vi "graph2.vi"(11 "replay":bool) -> (0 "path_size":i32, 3 "XY Graph":cluster{"Y":dbl[], "Y":dbl[]}[](graph)=[{"Y"=[-25.865695246715575, -25.865695246715575, -25.865695246715575], "Y"=[59.163033466791006, 59.163033466791006, 59.163033466791006]}, {"Y"=[0.85, 0.95, 0.95, 0.6, 0.6, 0.85, 0.85, -0.85, -0.85, -0.95, -0.95, -0.6, -0.6, -0.85, -0.6, -0.6, -0.85, -0.85, 0.85, 0.85], "Y"=[-0.6, -0.6, -1.4, -1.4, -0.6, -0.6, 2.4, 2.4, -0.6, -0.6, -1.4, -1.4, -0.6, -0.6, -0.6, -1.4, -1.4, -1.6, -1.6, -1.4]}, {"Y"=[-25.865695246715575], "Y"=[59.163033466791006]}, {"Y"=[], "Y"=[]}, {"Y"=array[926 elements], "Y"=array[926 elements]}, {"Y"=[nan, nan], "Y"=[nan, nan]}, {"Y"=[-25.865695246715575], "Y"=[59.163033466791006]}, {"Y"=[], "Y"=[]}, {"Y"=[], "Y"=[]}, {"Y"=[0.0], "Y"=[0.0]}, {"Y"=[], "Y"=[]}, {"Y"=[], "Y"=[]}, {"Y"=[691.7888277244315, 691.8377331659157, 691.8864790442867, 691.9350679862869, 691.9835025898547, 692.0317854247338, 692.079919033068, 692.1279059299806, 692.1757486041453, 692.2234495183519, 692.2710111100497, 692.3184357918904, 692.365725952261, 692.412883955801, 692.4599121439145, 692.5068128352747, 692.5535883263143, 692.6002408917145, 692.6467727848759, 692.6931862383941, 692.7394834645125, 692.785666655583, 692.8317379845035, 692.8776996051629, 692.9235536528688, 692.969302244769, 693.0149474802747, 693.060491441465, 693.1059361934975, 693.151283785001, 693.196536248471, 693.2416956006535, 693.2867638429291, 693.3317429616844, 693.3766349286853, 693.4214417014377, 693.4661652235502, 693.5108074250859, 693.5553702229134, 693.5998555210545, 693.6442652110193, 693.6886011721464, 693.7328652719325, 693.7770593663641, 693.8211853002351, 693.8652449074733, 693.9092400114525, 693.9531724253069, 693.9970439522381, 694.0408563858227, 694.0846115103164, 694.1283111009493, 694.1719569242241, 694.2155507382114, 694.259094292835, 694.3025893301664, 694.3460375847027, 694.3894407836557, 694.4328006472265, 694.476118888889, 694.5193972156585, 694.5626373283712, 694.6058409219545, 694.6490096856918, 694.6921453034947, 694.7352494541701, 694.7783238116778, 694.8213700453995, 694.8643898203949, 694.9073847976673, 694.9503566344149, 694.9933069842926, 695.0362374976652, 695.079149821865, 695.1220456014439, 695.1649264784243, 695.2077940925565, 695.2506500815632, 695.2934960813969, 695.3363337264864, 695.3791646499868, 695.4219904840265, 695.464812859962, 695.5076334086223, 695.5504537605557, 695.5932755462828, 695.6361003965429, 695.6789299425405, 695.7217658161954, 695.7646096503946, 695.807463079234, 695.8503277382761, 695.8932052647941, 695.9360972980251], "Y"=[-402.1714380892973, -402.2324443015287, -402.29325146963055, -402.3538628702814, -402.4142817442331, -402.47451129706894, -402.53455469993827, -402.5944150902866, -402.6540955725668, -402.71359921893855, -402.7729290699565, -402.832088135239, -402.8910793941361, -402.9499057963747, -403.00857026269705, -403.0670756854909, -403.12542492940014, -403.18362083193375, -403.24166620405737, -403.2995638307791, -403.3573164717253, -403.4149268617041, -403.4723977112591, -403.5297317072198, -403.58693151323575, -403.64399977030746, -403.7009390973042, -403.7577520914824, -403.81444132898264, -403.8710093653304, -403.9274587359257, -403.98379195652205, -404.0400115237071, -404.09611991536156, -404.1521195911291, -404.2080129928654, -404.2638025450895, -404.3194906554251, -404.375079715037, -404.4305720990579, -404.4859701670225, -404.5412762632748, -404.596492717394, -404.6516218445924, -404.70666594612766, -404.76162730969963, -404.81650820984265, -404.87131090831787, -404.9260376544974, -404.98069068574665, -405.0352722278018, -405.0897844951429, -405.14422969136206, -405.19861000952994, -405.2529276325616, -405.30718473357007, -405.3613834762236, -405.41552601510165, -405.46961449603776, -405.52365105647283, -405.5776378257941, -405.6315769256789, -405.685470470432, -405.7393205673213, -405.7931293169138, -405.84689881340205, -405.90063114494075, -405.9543283939694, -406.0079926375368, -406.0616259476311, -406.11523039149404, -406.1688080319476, -406.2223609277105, -406.2758911337184, -406.3294007014348, -406.38289167917463, -406.4363661124128, -406.4898260440976, -406.54327351496966, -406.5967105638653, -406.65013922803496, -406.70356154344927, -406.75697954511423, -406.8103952673769, -406.8638107442369, -406.9172280096572, -406.97064909787343, -407.0240760437018, -407.0775108828543, -407.1309556522436, -407.18441239029335, -407.23788313725817, -407.2913699355226, -407.3448748299264]}, {"Y"=[], "Y"=[]}, {"Y"=[-0.152017305614708], "Y"=[0.5451838106381299]}])   [LabVIEW 2015]
uses:
  G_NAV.vi
  G_PATH.vi
  G_VEH.vi
  G_SEN.vi
  G_LCM.vi
  <vilib>/Analysis/Matrix/Datatypes/RealMatrix.ctl
  <vilib>/Analysis/Matrix/NI_Matrix.lvlib
  <vilib>/Analysis/NI_AALBase.lvlib
  <vilib>/Analysis/baseanly.llb/Real A x B.vi
panel:
  out "x 17":dbl[](array[numeric])=[-13.0, -13.0, -13.0, -13.0, -13.0, -13.0, -13.0, -13.0, -13.0, -13.0, -13.0, -13.0, -13.0, -13.0, -13.0, -13.0, -13.0, -13.0, -13.0, -13.0, -13.0, -13.0, -13.0, -13.0, -13.0, -13.25, -13.25, -13.25, -13.25, -13.25, -13.25, -13.25, -13.25, -13.25, -13.25, -13.25, -13.25, -13.25, -13.25, -13.25, -13.25, -13.25, -13.25, -13.25, -13.25, -13.5, -13.25, -13.25, -13.25, -13.5, -13.5, -13.25, -13.5, -13.5, -13.5, -13.5, -13.5, -13.25, -13.5, -13.5, -13.75, -13.5, -13.5, -13.25, -13.75, -13.75, -13.5, -13.5, -13.5, -14.0, -14.0, -14.0, -13.75, -13.75, -13.75, -13.75, -1.0, -1.0, -0.75, -0.75, -0.75, -0.5, -0.5, -0.5, -0.25, -0.25, -0.25, -0.25, 0.0, 0.0, 0.0, 0.0, 0.0, 0.25, 0.25, 0.25, 0.25, 0.25, 0.5, 0.5, 0.5, 0.5, 0.75, 0.75, 0.75, 1.0, 1.0, 1.25, 1.25, 1.25, 1.5, 1.5]
  out "y 17":dbl[](array[numeric])=[0.0, 0.25, 0.5, 0.75, 1.0, 1.25, 1.25, 1.5, 1.75, 2.0, 2.25, 2.5, 2.75, 3.0, 3.25, 3.5, 3.75, 4.0, 4.25, 4.5, 4.75, 5.0, 5.25, 5.5, 5.75, 6.0, 6.5, 6.75, 7.0, 7.25, 7.5, 8.0, 8.25, 8.5, 9.0, 9.25, 9.5, 10.0, 10.25, 10.75, 11.25, 11.5, 12.0, 12.5, 13.0, 13.5, 13.75, 14.25, 14.75, 15.5, 16.0, 16.5, 17.25, 18.0, 18.5, 19.5, 20.0, 20.5, 21.75, 22.25, 23.75, 24.5, 25.25, 26.25, 28.25, 29.25, 30.5, 31.75, 33.25, 36.5, 38.25, 40.5, 42.75, 45.25, 48.25, 51.5, 4.25, 4.0, 4.0, 4.0, 3.75, 3.75, 3.75, 3.5, 3.5, 3.5, 3.25, 3.25, 3.25, 3.25, 3.25, 3.25, 3.0, 3.0, 3.0, 3.0, 3.0, 2.75, 3.0, 3.0, 3.0, 3.25, 3.25, 3.25, 3.5, 3.5, 3.5, 3.75, 3.75, 4.0, 4.0, 4.25]
  out "x 16":dbl[](array[numeric])=[-13.0, -13.0, -13.0, -13.0, -13.0, -13.0, -13.0, -13.0, -13.0, -13.0, -13.0, -13.0, -13.0, -13.0, -13.0, -13.0, -13.0, -13.0, -13.0, -13.0, -13.0, -13.0, -13.0, -13.0, -13.0, -13.25, -13.25, -13.25, -13.25, -13.25, -13.25, -13.25, -13.25, -13.25, -13.25, -13.25, -13.25, -13.25, -13.25, -13.25, -13.25, -13.25, -13.25, -13.25, -13.25, -13.5, -13.25, -13.25, -13.25, -13.5, -13.5, -13.25, -13.5, -13.5, -13.5, -13.5, -13.5, -13.25, -13.5, -13.5, -13.75, -13.5, -13.5, -13.25, -13.75, -13.75, -13.5, -13.5, -13.5, -14.0, -14.0, -14.0, -13.75, -13.75, -13.75, -13.75, -1.0, -1.0, -0.75, -0.75, -0.75, -0.5, -0.5, -0.5, -0.25, -0.25, -0.25, -0.25, 0.0, 0.0, 0.0, 0.0, 0.0, 0.25, 0.25, 0.25, 0.25, 0.25, 0.5, 0.5, 0.5, 0.5, 0.75, 0.75, 0.75, 1.0, 1.0, 1.25, 1.25, 1.25, 1.5, 1.5]
  out "y 16":dbl[](array[numeric])=[0.0, 0.25, 0.5, 0.75, 1.0, 1.25, 1.25, 1.5, 1.75, 2.0, 2.25, 2.5, 2.75, 3.0, 3.25, 3.5, 3.75, 4.0, 4.25, 4.5, 4.75, 5.0, 5.25, 5.5, 5.75, 6.0, 6.5, 6.75, 7.0, 7.25, 7.5, 8.0, 8.25, 8.5, 9.0, 9.25, 9.5, 10.0, 10.25, 10.75, 11.25, 11.5, 12.0, 12.5, 13.0, 13.5, 13.75, 14.25, 14.75, 15.5, 16.0, 16.5, 17.25, 18.0, 18.5, 19.5, 20.0, 20.5, 21.75, 22.25, 23.75, 24.5, 25.25, 26.25, 28.25, 29.25, 30.5, 31.75, 33.25, 36.5, 38.25, 40.5, 42.75, 45.25, 48.25, 51.5, 4.25, 4.0, 4.0, 4.0, 3.75, 3.75, 3.75, 3.5, 3.5, 3.5, 3.25, 3.25, 3.25, 3.25, 3.25, 3.25, 3.0, 3.0, 3.0, 3.0, 3.0, 2.75, 3.0, 3.0, 3.0, 3.25, 3.25, 3.25, 3.5, 3.5, 3.5, 3.75, 3.75, 4.0, 4.0, 4.25]
  out "M6006":T1={"GPSTime"=22892800.0, "attitude[2]"=-0.6123908, "lcc[0]"=-970.47205, "lcc[1]"=200.52362, "heading_GPS"=-0.6106907} {"GPSTime" format="%#_6f"}
  out "y 5":dbl[](array[numeric])
  out "x 5":dbl[](array[numeric])
  out "y 4":dbl[](array[numeric])
  out "x 4":dbl[](array[numeric])
  out "y 6":dbl[](array[numeric])
  out "x 6":dbl[](array[numeric])
  out "x 14":dbl[](array[numeric])
  out "y 14":dbl[](array[numeric])
  out "y 10":dbl[](array[numeric])
  out "x 10":dbl[](array[numeric])
  out "y 1":dbl[](array[numeric])
  out "x 1":dbl[](array[numeric])
  out "y 15":dbl[](array[numeric])=[0.0, 0.25, 0.5, 0.75, 1.0, 1.25, 1.25, 1.5, 1.75, 2.0, 2.25, 2.5, 2.75, 3.0, 3.25, 3.5, 3.75, 4.0, 4.25, 4.5, 4.75, 5.0, 5.25, 5.5, 5.75, 6.0, 6.5, 6.75, 7.0, 7.25, 7.5, 8.0, 8.25, 8.5, 9.0, 9.25, 9.5, 10.0, 10.25, 10.75, 11.25, 11.5, 12.0, 12.5, 13.0, 13.5, 13.75, 14.25, 14.75, 15.5, 16.0, 16.5, 17.25, 18.0, 18.5, 19.5, 20.0, 20.5, 21.75, 22.25, 23.75, 24.5, 25.25, 26.25, 28.25, 29.25, 30.5, 31.75, 33.25, 36.5, 38.25, 40.5, 42.75, 45.25, 48.25, 51.5, 4.25, 4.0, 4.0, 4.0, 3.75, 3.75, 3.75, 3.5, 3.5, 3.5, 3.25, 3.25, 3.25, 3.25, 3.25, 3.25, 3.0, 3.0, 3.0, 3.0, 3.0, 2.75, 3.0, 3.0, 3.0, 3.25, 3.25, 3.25, 3.5, 3.5, 3.5, 3.75, 3.75, 4.0, 4.0, 4.25]
  out "x 15":dbl[](array[numeric])=[-13.0, -13.0, -13.0, -13.0, -13.0, -13.0, -13.0, -13.0, -13.0, -13.0, -13.0, -13.0, -13.0, -13.0, -13.0, -13.0, -13.0, -13.0, -13.0, -13.0, -13.0, -13.0, -13.0, -13.0, -13.0, -13.25, -13.25, -13.25, -13.25, -13.25, -13.25, -13.25, -13.25, -13.25, -13.25, -13.25, -13.25, -13.25, -13.25, -13.25, -13.25, -13.25, -13.25, -13.25, -13.25, -13.5, -13.25, -13.25, -13.25, -13.5, -13.5, -13.25, -13.5, -13.5, -13.5, -13.5, -13.5, -13.25, -13.5, -13.5, -13.75, -13.5, -13.5, -13.25, -13.75, -13.75, -13.5, -13.5, -13.5, -14.0, -14.0, -14.0, -13.75, -13.75, -13.75, -13.75, -1.0, -1.0, -0.75, -0.75, -0.75, -0.5, -0.5, -0.5, -0.25, -0.25, -0.25, -0.25, 0.0, 0.0, 0.0, 0.0, 0.0, 0.25, 0.25, 0.25, 0.25, 0.25, 0.5, 0.5, 0.5, 0.5, 0.75, 0.75, 0.75, 1.0, 1.0, 1.25, 1.25, 1.25, 1.5, 1.5]
  out "y 13":dbl[](array[numeric])=[0.0, 0.25, 0.5, 0.75, 1.0, 1.25, 1.25, 1.5, 1.75, 2.0, 2.25, 2.5, 2.75, 3.0, 3.25, 3.5, 3.75, 4.0, 4.25, 4.5, 4.75, 5.0, 5.25, 5.5, 5.75, 6.0, 6.5, 6.75, 7.0, 7.25, 7.5, 8.0, 8.25, 8.5, 9.0, 9.25, 9.5, 10.0, 10.25, 10.75, 11.25, 11.5, 12.0, 12.5, 13.0, 13.5, 13.75, 14.25, 14.75, 15.5, 16.0, 16.5, 17.25, 18.0, 18.5, 19.5, 20.0, 20.5, 21.75, 22.25, 23.75, 24.5, 25.25, 26.25, 28.25, 29.25, 30.5, 31.75, 33.25, 36.5, 38.25, 40.5, 42.75, 45.25, 48.25, 51.5, 4.25, 4.0, 4.0, 4.0, 3.75, 3.75, 3.75, 3.5, 3.5, 3.5, 3.25, 3.25, 3.25, 3.25, 3.25, 3.25, 3.0, 3.0, 3.0, 3.0, 3.0, 2.75, 3.0, 3.0, 3.0, 3.25, 3.25, 3.25, 3.5, 3.5, 3.5, 3.75, 3.75, 4.0, 4.0, 4.25]
  out "x 13":dbl[](array[numeric])=[-13.0, -13.0, -13.0, -13.0, -13.0, -13.0, -13.0, -13.0, -13.0, -13.0, -13.0, -13.0, -13.0, -13.0, -13.0, -13.0, -13.0, -13.0, -13.0, -13.0, -13.0, -13.0, -13.0, -13.0, -13.0, -13.25, -13.25, -13.25, -13.25, -13.25, -13.25, -13.25, -13.25, -13.25, -13.25, -13.25, -13.25, -13.25, -13.25, -13.25, -13.25, -13.25, -13.25, -13.25, -13.25, -13.5, -13.25, -13.25, -13.25, -13.5, -13.5, -13.25, -13.5, -13.5, -13.5, -13.5, -13.5, -13.25, -13.5, -13.5, -13.75, -13.5, -13.5, -13.25, -13.75, -13.75, -13.5, -13.5, -13.5, -14.0, -14.0, -14.0, -13.75, -13.75, -13.75, -13.75, -1.0, -1.0, -0.75, -0.75, -0.75, -0.5, -0.5, -0.5, -0.25, -0.25, -0.25, -0.25, 0.0, 0.0, 0.0, 0.0, 0.0, 0.25, 0.25, 0.25, 0.25, 0.25, 0.5, 0.5, 0.5, 0.5, 0.75, 0.75, 0.75, 1.0, 1.0, 1.25, 1.25, 1.25, 1.5, 1.5]
  out "y 12":dbl[](array[numeric])=[0.0, 0.25, 0.5, 0.75, 1.0, 1.25, 1.25, 1.5, 1.75, 2.0, 2.25, 2.5, 2.75, 3.0, 3.25, 3.5, 3.75, 4.0, 4.25, 4.5, 4.75, 5.0, 5.25, 5.5, 5.75, 6.0, 6.5, 6.75, 7.0, 7.25, 7.5, 8.0, 8.25, 8.5, 9.0, 9.25, 9.5, 10.0, 10.25, 10.75, 11.25, 11.5, 12.0, 12.5, 13.0, 13.5, 13.75, 14.25, 14.75, 15.5, 16.0, 16.5, 17.25, 18.0, 18.5, 19.5, 20.0, 20.5, 21.75, 22.25, 23.75, 24.5, 25.25, 26.25, 28.25, 29.25, 30.5, 31.75, 33.25, 36.5, 38.25, 40.5, 42.75, 45.25, 48.25, 51.5, 4.25, 4.0, 4.0, 4.0, 3.75, 3.75, 3.75, 3.5, 3.5, 3.5, 3.25, 3.25, 3.25, 3.25, 3.25, 3.25, 3.0, 3.0, 3.0, 3.0, 3.0, 2.75, 3.0, 3.0, 3.0, 3.25, 3.25, 3.25, 3.5, 3.5, 3.5, 3.75, 3.75, 4.0, 4.0, 4.25]
  out "x 12":dbl[](array[numeric])=[-13.0, -13.0, -13.0, -13.0, -13.0, -13.0, -13.0, -13.0, -13.0, -13.0, -13.0, -13.0, -13.0, -13.0, -13.0, -13.0, -13.0, -13.0, -13.0, -13.0, -13.0, -13.0, -13.0, -13.0, -13.0, -13.25, -13.25, -13.25, -13.25, -13.25, -13.25, -13.25, -13.25, -13.25, -13.25, -13.25, -13.25, -13.25, -13.25, -13.25, -13.25, -13.25, -13.25, -13.25, -13.25, -13.5, -13.25, -13.25, -13.25, -13.5, -13.5, -13.25, -13.5, -13.5, -13.5, -13.5, -13.5, -13.25, -13.5, -13.5, -13.75, -13.5, -13.5, -13.25, -13.75, -13.75, -13.5, -13.5, -13.5, -14.0, -14.0, -14.0, -13.75, -13.75, -13.75, -13.75, -1.0, -1.0, -0.75, -0.75, -0.75, -0.5, -0.5, -0.5, -0.25, -0.25, -0.25, -0.25, 0.0, 0.0, 0.0, 0.0, 0.0, 0.25, 0.25, 0.25, 0.25, 0.25, 0.5, 0.5, 0.5, 0.5, 0.75, 0.75, 0.75, 1.0, 1.0, 1.25, 1.25, 1.25, 1.5, 1.5]
  out "y 11":dbl[](array[numeric])=[0.0, 0.25, 0.5, 0.75, 1.0, 1.25, 1.25, 1.5, 1.75, 2.0, 2.25, 2.5, 2.75, 3.0, 3.25, 3.5, 3.75, 4.0, 4.25, 4.5, 4.75, 5.0, 5.25, 5.5, 5.75, 6.0, 6.5, 6.75, 7.0, 7.25, 7.5, 8.0, 8.25, 8.5, 9.0, 9.25, 9.5, 10.0, 10.25, 10.75, 11.25, 11.5, 12.0, 12.5, 13.0, 13.5, 13.75, 14.25, 14.75, 15.5, 16.0, 16.5, 17.25, 18.0, 18.5, 19.5, 20.0, 20.5, 21.75, 22.25, 23.75, 24.5, 25.25, 26.25, 28.25, 29.25, 30.5, 31.75, 33.25, 36.5, 38.25, 40.5, 42.75, 45.25, 48.25, 51.5, 4.25, 4.0, 4.0, 4.0, 3.75, 3.75, 3.75, 3.5, 3.5, 3.5, 3.25, 3.25, 3.25, 3.25, 3.25, 3.25, 3.0, 3.0, 3.0, 3.0, 3.0, 2.75, 3.0, 3.0, 3.0, 3.25, 3.25, 3.25, 3.5, 3.5, 3.5, 3.75, 3.75, 4.0, 4.0, 4.25]
  out "x 11":dbl[](array[numeric])=[-13.0, -13.0, -13.0, -13.0, -13.0, -13.0, -13.0, -13.0, -13.0, -13.0, -13.0, -13.0, -13.0, -13.0, -13.0, -13.0, -13.0, -13.0, -13.0, -13.0, -13.0, -13.0, -13.0, -13.0, -13.0, -13.25, -13.25, -13.25, -13.25, -13.25, -13.25, -13.25, -13.25, -13.25, -13.25, -13.25, -13.25, -13.25, -13.25, -13.25, -13.25, -13.25, -13.25, -13.25, -13.25, -13.5, -13.25, -13.25, -13.25, -13.5, -13.5, -13.25, -13.5, -13.5, -13.5, -13.5, -13.5, -13.25, -13.5, -13.5, -13.75, -13.5, -13.5, -13.25, -13.75, -13.75, -13.5, -13.5, -13.5, -14.0, -14.0, -14.0, -13.75, -13.75, -13.75, -13.75, -1.0, -1.0, -0.75, -0.75, -0.75, -0.5, -0.5, -0.5, -0.25, -0.25, -0.25, -0.25, 0.0, 0.0, 0.0, 0.0, 0.0, 0.25, 0.25, 0.25, 0.25, 0.25, 0.5, 0.5, 0.5, 0.5, 0.75, 0.75, 0.75, 1.0, 1.0, 1.25, 1.25, 1.25, 1.5, 1.5]
  out "y 9":dbl[](array[numeric])=[-40.25486400827094, -40.04085960963455, -39.821235299880705, -39.59593792545196, -39.364914332790825, -39.12811136833988, -38.88547587854164, -38.636954709838655, -38.382494708673484, -38.12204272148863, -37.85554559472668, -37.58295017483014, -37.30420330824157, -37.0192518414035, -36.728042620758494, -36.43052249274907, -36.126638303817785, -35.81633690040717, -35.49956512895978, -35.176269835918156, -34.846397867724825, -34.50989607082233, -34.166711291653236, -33.81679037666006, -33.460080172285366, -33.09652752497168, -32.72607928116154, -32.3486822872975, -31.96428338982209, -31.57282943517787, -31.17426726980736, -30.768543740153135, -30.355605692657697, -30.338651341222633, -30.338651341222633, -29.95729378436619, -29.572397676750224, -29.183911226613308, -28.791782642194068, -28.395960131731087, -27.996391903462964, -27.593026165628288, -27.185811126465662, -26.774694994213668, -26.359625977110902, -25.940552283395995, -25.5174221213075, -25.090183699084033, -24.658785224964184, -24.22317490718656, -23.783300953989748, -23.33911157361234, -22.89055497429293, -22.43757936427013, -21.980132951782515, -21.5181639450687, -21.05162055236726, -20.58045098191681, -20.10460344195595, -19.62402614072324, -19.138667286457324, -18.648475087396758, -18.153397751780158, -17.653383487846114, -17.14838050383323, -16.6383370079801, -16.123201208525305, -15.602921313707439, -15.077445531765132, -14.546722070936944, -14.010699139461483, -13.469324945577348, -12.922547697523145, -12.370315603537431, -11.812576871858855, -11.249279710725965, -10.68037232837739, -10.105802933051706, -9.52551973298753, -8.939470936423437, -8.347604751598034, -8.312579060465806, -8.312579060465806, -7.815979397588906, -7.318560473773825, -6.820356240811432, -6.321400650492564, -5.8217276546080905, -5.321371204948849, -4.820365253305692, -4.318743751469474, -3.816540651231034, -3.313789904381253, -2.8105254627109564, -2.3067812780109964, -1.8025913020722415, -1.2979894866855162, -0.7930097836417018, -0.2876861447316371, 0.2179474782538381, 0.7238571335238572, 1.2300088692875666, 1.7363687337541345, 2.2429027751326935, 2.7495770416323975, 3.2563575814623866, 3.763210442831828, 4.270101673949855, 4.776997323025622, 5.283863438268267, 5.79066606788696, 6.297371260090832, 6.803945063089038, 7.310353525090725, 7.816562694305046, 8.322538618941149, 8.82824734720817, 9.333654927315276, 9.532792066869051, 9.532792066869058, 10.032676667529001, 10.532532309358876, 11.032359899557544, 11.53216034532386, 12.03193455385667, 12.53168343235485, 13.03140788801724, 13.531108828042706, 14.030787159630101, 14.530443789978285, 15.030079626286113, 15.529695575752449, 16.029292545576137, 16.52887144295605, 17.028433175091028, 17.527978649179936, 18.02750877242164, 18.527024452014977, 19.026526595158828, 19.526016109052026, 20.025493900893448, 20.52496087788194, 21.02441794721636, 21.523866016095567, 22.023305991718424, 22.522738781283774, 23.022165291990486, 23.521586431037413, 24.021003105623414, 24.520416222947343, 25.01982669020806, 25.51923541460442, 26.018643303335274, 26.518051263599492, 27.017460202595917, 27.51687102752342, 28.016284645580857, 28.515701963967068, 29.01512388988093, 29.51455133052128, 30.013985193087, 30.513426384776935, 31.012875812789932, 31.512334384324856, 32.01180300658057, 32.511282586755925, 33.01077403204978, 33.51027824966099, 34.00979614678842, 34.15163746485512, 34.15163746485511, 34.65085156194158, 35.150114036225105, 35.649423358614406, 36.148778000018126, 36.64817643134495, 37.14761712350358, 37.64709854740265, 38.14661917395086, 38.64617747405689, 39.14577191862942, 39.6454009785771, 40.14506312480863, 40.644756828232666, 41.14448055975791, 41.644232790293024, 42.14401199074667, 42.643816632027544, 43.14364518504432, 43.64349612070567, 44.14336790992027, 44.6432590235968, 45.14316793264393, 45.64309310797034, 46.143033020484694, 46.64298614109569, 47.14295094071199, 47.64292589024228, 48.14290946059522, 48.64290012267951, 49.142896347403784, 49.64289660567677, 50.142899368407114, 50.64290310650349, 51.14290629087459, 51.64290739242908, 52.14290488207564, 52.64289723072293, 53.142882909279656, 53.642860388654476, 54.14282813975608, 54.64278463349311, 55.14272834077427, 55.64265773250823, 56.14257127960367, 56.642467452969264, 57.142344723513695, 57.642201562145615, 58.14203643977374, 58.6418478273067, 59.141634195653204, 59.641394015721914, 60.1411257584215, 60.64082789466066, 61.14049889534806, 61.64013723139237, 62.139741373702265, 62.63930979318643, 63.138840960753534, 63.63833334731226, 64.13778542377129, 64.63719566103929, 65.1365625300249, 65.63588450163687, 66.13516004678382, 66.62661681170006, 66.62661681170006, 67.12576345342403, 67.62478981859165, 68.1236869902195, 68.62244605132406, 69.12105808492187, 69.61951417402948, 70.11780540166339, 70.61592285084015, 71.11385760457627, 71.61160074588827, 72.10914335779272, 72.6064765233061, 73.10359132544497, 73.60047884722584, 74.09713017166524, 74.59353638177971, 75.08968856058576, 75.58557779109994, 76.08119515633875, 76.57653173931875, 77.07157862305642, 77.56632689056836, 78.060767624871, 78.55489190898098, 79.04869082591473, 79.54215545868882, 80.03527689031979, 80.52804620382416, 81.02045448221844, 81.51249280851917, 82.00415226574289, 82.49542393690609, 82.98629890502534, 83.47676825311716, 83.96682306419804, 84.45645442128455, 84.9456534073932, 85.43441110554052, 85.92271859874306, 86.4105669700173, 86.89794730237979, 87.17622393756727, 87.17622393756727, 87.62090998324233, 88.06278904034333, 88.5018353078985, 88.93802298493607, 89.37132627048422, 89.80171936357122, 90.22917646322526, 90.65367176847454, 91.07517947834734, 91.49367379187183, 91.90912890807624, 92.3215190259888, 92.73081834463773, 93.13700106305124, 93.54004138025758, 93.93991349528491, 94.3365916071615, 94.73004991491554, 95.12026261757528, 95.50720391416891, 95.89084800372467, 96.27116908527078, 96.64814135783546, 97.02173902044692, 97.39193627213336, 97.75870731192305, 98.12202633884417, 98.48186755192496, 98.83820515019363, 99.19101333267841, 99.54026629840749, 99.88593824640913, 99.89953643323281, 99.89953643323281, 100.21054094201504, 100.51734678566943, 100.81989169992012, 101.11811342049135, 101.41194968310735, 101.70133822349231, 101.98621677737043, 102.26652308046596, 102.54219486850307, 102.81316987720602, 103.07938584229896, 103.34078049950615, 103.59729158455178, 103.84885683316006, 104.09541398105519, 104.33690076396141, 104.5732549176029, 104.80441417770389, 105.0303162799886, 105.2508989601812, 105.46609995400595, 105.67585699718703, 105.88010782544866, 106.07879017451506, 106.27184178011042, 106.45920037795898, 106.64080370378494, 106.81658949331246, 106.98649548226584, 107.15045940636924, 107.30841900134685, 107.46031200292295, 107.60607614682168, 107.74564916876727, 107.87896880448396, 108.00597278969595, 108.12659886012742, 108.24078475150262, 108.34846819954572, 108.44958693998096, 108.54407870853257, 108.63188124092471, 108.71293227288164, 108.78716954012754, 108.85453077838663, 108.91495372338314, 108.96837611084122, 108.97747618937277, 108.97747618937277, 109.0156550246946, 109.04983247580746, 109.08011123358501, 109.10659398890081, 109.12938343262847, 109.14858225564154, 109.16429314881364, 109.17661880301837, 109.18566190912927, 109.19152515801999, 109.19431124056405, 109.19412284763511, 109.1910626701067, 109.18523339885247, 109.17673772474595, 109.16567833866077, 109.15215793147051, 109.13627919404871, 109.11814481726906, 109.09785749200506, 109.07551990913035, 109.05123475951848, 109.02510473404305, 108.99723252357771, 108.96772081899594, 108.93667231117144, 108.90418969097772, 108.87037564928839, 108.83533287697705, 108.79916406491728, 108.7619719039827, 108.72385908504685, 108.68492829898334, 108.64528223666576, 108.60502358896771, 108.56425504676278, 108.52307930092454, 108.48159904232658, 108.4399169618425, 108.39813575034592, 108.35635809871036, 108.31468669780945, 108.27322423851678, 108.23207341170594, 108.19133690825049, 108.15111741902408, 108.11151763490025, 108.07264024675257, 108.03458794545469, 107.99746342188017, 107.96136936690259, 107.92640847139555, 107.89268342623265, 107.86029692228745, 107.82935165043357, 107.79995030154457, 107.78125898031978, 107.78125898031978, 107.75369240153198, 107.72548456275034, 107.69669916249154, 107.66739989927227, 107.63765047160923, 107.60751457801909, 107.57705591701853, 107.54633818712422, 107.51542508685286, 107.48438031472112, 107.45326756924571, 107.42215054894329, 107.39109295233057, 107.36015847792419, 107.32941082424084, 107.29891368979723, 107.26873077311004, 107.23892577269594, 107.2095623870716, 107.18070431475374, 107.15241525425903, 107.12475890410411, 107.09779896280573, 107.07159912888052, 107.04622310084521, 107.02173457721644, 106.9981972565109, 106.97567483724531, 106.95423101793631, 106.9339294971006, 106.91483397325487, 106.89700814491579, 106.88051571060006, 106.86545285263342, 106.86545285263342, 106.85123591176482, 106.8373215059327, 106.82369194296759, 106.81032953069995, 106.79721657696027, 106.78433538957903, 106.7716682763867, 106.75919754521381, 106.74690550389077, 106.73477446024813, 106.72278672211637, 106.71092459732593, 106.69917039370733, 106.68750641909104, 106.67591498130754, 106.66437838818732, 106.65287894756085, 106.64139896725864, 106.62992075511116, 106.61842661894889, 106.60689886660232, 106.59531980590192, 106.5836717446782, 106.57193699076163, 106.56009785198269, 106.54813663617186, 106.53603565115962, 106.52377720477648, 106.51134360485288, 106.49871715921937, 106.4858801757064, 106.47281496214443, 106.45950382636393, 106.44592907619545, 106.43207301946944, 106.41791796401637, 106.40344621766674, 106.38864008825105, 106.37348188359975, 106.35795391154335, 106.34203847991229, 106.32571789653713, 106.30897446924827, 106.29179050587625, 106.27414831425155, 106.2560637066309]
  out "x 9":dbl[](array[numeric])=[-22.968902627554595, -22.51700484334325, -22.067726202847595, -21.62109147813308, -21.177125441265126, -20.735852864309198, -20.297298519330727, -19.86148717839516, -19.42844361356793, -18.998192596914485, -18.57075890050028, -18.146167296390736, -17.724442556651315, -17.305609453347444, -16.889692758544577, -16.476717244308148, -16.0667076827036, -15.659688845796383, -15.255685505651932, -14.854722434335699, -14.456824403913117, -14.062016186449632, -13.67032255401068, -13.28176827866172, -12.896378132468183, -12.514176887495505, -12.135189315809143, -11.759440189474532, -11.38695428055711, -11.017756361122329, -10.651871203235629, -10.289323578962446, -9.930138260368233, -9.915595940630572, -9.915595940630572, -9.592217431479307, -9.27296664733781, -8.957904003376973, -8.64708991476769, -8.340584796680856, -8.038449064287356, -7.740743132758091, -7.447527417263952, -7.158862332975826, -6.874808295064605, -6.595425718701188, -6.320775019056462, -6.05091661130132, -5.7859109106066535, -5.525818332143363, -5.270699291082332, -5.02061420259445, -4.775623481850621, -4.535787544021732, -4.301166804278667, -4.071821677792334, -3.8478125797336116, -3.6291999252734, -3.4160441295825903, -3.2084056078320766, -3.0063447751927437, -2.809922046835485, -2.619197837931207, -2.4342325636507813, -2.255086639165114, -2.0818204796450988, -1.9144945002616136, -1.7531691161855663, -1.597904742587841, -1.4487617946393383, -1.3058006875109367, -1.1690818363735358, -1.0386656563980352, -0.9146125627553217, -0.796982970616279, -0.6858372951518088, -0.581235951532802, -0.4832393549301528, -0.3919079205147527, -0.30730206345748806, -0.22948219892925836, -0.22511372738602808, -0.22511372738602808, -0.16680067513880384, -0.11507613036628858, -0.06966705231019729, -0.03030040021222455, 0.0032968666859287954, 0.03139778914256819, 0.05427540791599236, 0.07220276376450722, 0.08545289744639678, 0.09429884971998208, 0.09901366134354672, 0.09987037307539658, 0.09714202567383796, 0.0911016598971616, 0.08202231650367428, 0.0701770362516814, 0.055838859899467026, 0.0392808282053517, 0.020775981927619973, 0.0005973618245841139, -0.020981991345463767, -0.043689036824225154, -0.06725073385338684, -0.09139404167465787, -0.11584591952973904, -0.14033332666033183, -0.164583222308123, -0.18832256571482164, -0.21127831612212852, -0.233177432771738, -0.25374687490535136, -0.27271360176467, -0.28980457259138814, -0.30474674662721396, -0.31726708311384183, -0.32147712013105156, -0.3214771201310518, -0.3322441522303675, -0.3444544578596952, -0.3580628233106866, -0.37302403487498664, -0.38929287884424707, -0.4068241415101202, -0.4255726091642576, -0.44549306809831846, -0.4665403046039335, -0.4886691049727688, -0.5118342554964762, -0.5359905424667011, -0.5610927521750875, -0.5870956709133022, -0.6139540849729826, -0.6416227806457879, -0.670056544223363, -0.6992101619973595, -0.72903842025943, -0.7594961053012258, -0.7905380034143993, -0.8221189008906022, -0.8541935840214723, -0.8867168390986828, -0.9196434524138646, -0.9529282102586762, -0.9865258989247632, -1.0203913047037911, -1.0544792138873982, -1.088744412767236, -1.1231416876349567, -1.1576258247822122, -1.192151610500654, -1.2266738310819347, -1.261147272817699, -1.2955267219995985, -1.329766964919293, -1.3638227878684193, -1.3976489771386371, -1.4312003190215978, -1.4644315998089543, -1.4972976057923506, -1.5297531232634387, -1.5617529385138709, -1.593251837835299, -1.6242046075193748, -1.6545660338577437, -1.684290903142064, -1.713334001663981, -1.7214502693093892, -1.721450269309389, -1.7494765704663608, -1.7766543195019637, -1.803010337186423, -1.8285714442899548, -1.8533644615827702, -1.8774162098350855, -1.9007535098171258, -1.9234031822991002, -1.9453920480512341, -1.966746927843737, -1.9874946424468334, -2.00766201263074, -2.027275859165667, -2.046363002821832, -2.0649502643694664, -2.083064464578773, -2.1007324242199688, -2.1179809640632783, -2.1348369048789184, -2.1513270674370997, -2.1674782725080464, -2.183317340861975, -2.198871093269103, -2.2141663504996414, -2.229229933323813, -2.244088662511829, -2.2587693588339204, -2.27329884306029, -2.2877039359611624, -2.3020114583067546, -2.316248230867277, -2.3304410744129536, -2.3446168097140014, -2.358802257540638, -2.3730242386630804, -2.387309573851546, -2.401685083876244, -2.4161775895074067, -2.430813911515237, -2.445620870669959, -2.46062528774179, -2.4758539835009468, -2.491333778717647, -2.5070914941621076, -2.523153950604546, -2.539547968815179, -2.556300369564224, -2.573437973621899, -2.5909876017584192, -2.6089760747440036, -2.6274302133488687, -2.646376838343232, -2.66584277049731, -2.68585483058132, -2.7064398393654807, -2.7276246176200143, -2.749435986115125, -2.7719007656210435, -2.7950457769079735, -2.818897840746146, -2.843483777905771, -2.8688304091570727, -2.8949645552702545, -2.921913037015548, -2.9492635082994942, -2.9492635082994942, -2.978480917327609, -3.0098270674333767, -3.043459777809386, -3.079536867648219, -3.118216156142463, -3.1596554624846984, -3.204012605867507, -3.2514454054834765, -3.3021116805251873, -3.3561692501852223, -3.4137759336561606, -3.4750895501305976, -3.5402679188011072, -3.6094688588602786, -3.682850189500691, -3.760569729914927, -3.842785299295573, -3.929654716835212, -4.021335801726423, -4.117986373161795, -4.219764250333915, -4.326827252435352, -4.439333198658707, -4.557439908196553, -4.6813052002414715, -4.811086893986051, -4.946942808622881, -5.089030763344532, -5.237508577343594, -5.392534069812648, -5.554265059944274, -5.722859366931069, -5.898474809965605, -6.081269208240471, -6.27140038094824, -6.469026147281509, -6.674304326432857, -6.88739273759486, -7.10844919996011, -7.33763153272119, -7.5750975550706805, -7.714565866361133, -7.714565866361133, -7.943178762901428, -8.177335605648189, -8.417087352842183, -8.6624849627242, -8.913579393535008, -9.170421603515402, -9.433062550906158, -9.701553193948051, -9.975944490881862, -10.256287399948372, -10.542632879388364, -10.835031887442614, -11.133535382351901, -11.438194322357017, -11.74905966569872, -12.06618237061781, -12.389613395355056, -12.719403698151243, -13.055604237247149, -13.398265970883559, -13.747439857301249, -14.10317685474099, -14.465527921443577, -14.83454401564979, -15.210276095600387, -15.592775119536174, -15.982092045697918, -16.378277832326408, -16.78138343766241, -17.19145981994672, -17.608557937420102, -18.032728748323343, -18.0496518526286, -18.0496518526286, -18.441165968034287, -18.83605201755941, -19.234360005438532, -19.636139935906236, -20.041441813197096, -20.450315641545686, -20.862811425186578, -21.278979168354343, -21.698868875283566, -22.122530550208822, -22.550014197364675, -22.98136982098571, -23.41664742530649, -23.8558970145616, -24.29916859298561, -24.746512164813097, -25.197977734278638, -25.6536153056168, -26.113474883062164, -26.5776064708493, -27.046060073212793, -27.5188856943872, -27.996133338607113, -28.4778530101071, -28.96409471312173, -29.454908451885586, -29.950344230633245, -30.450452053599268, -30.95528192501824, -31.46488384912474, -31.979307830153324, -32.49860387233859, -33.0228219799151, -33.552012157117424, -34.08622440818015, -34.625508737337846, -35.16991514882508, -35.719493646876444, -36.2742942357265, -36.83436691960981, -37.39976170276098, -37.97052858941455, -38.54671758380513, -39.12837869016727, -39.71556191273555, -40.308317255744555, -40.90669472342885, -41.01788165020217, -41.01788165020217, -41.516426075908484, -42.01529336894664, -42.514475243301945, -43.01396341295969, -43.51374959190518, -44.013825494123736, -44.514182833600636, -45.01481332432121, -45.515708680270734, -46.01686061543453, -46.51826084379791, -47.019901079346155, -47.521773036064594, -48.0238684279385, -48.526178968953204, -49.02869637309399, -49.53141235434619, -50.03431862669508, -50.53740690412599, -51.04066890062418, -51.54409633017501, -52.04768090676373, -52.55141434437569, -53.055288356996165, -53.55929465861046, -54.0634249632039, -54.56767098476177, -55.072024437269384, -55.576477034712035, -56.08102049107504, -56.58564652034369, -57.090346836503294, -57.59511315353915, -58.09993718543659, -58.60481064618088, -59.109725249757346, -59.61467271015128, -60.119644741348004, -60.62463305733281, -61.129629372090996, -61.63462539960787, -62.13961285386874, -62.64458344885892, -63.149528898563695, -63.65444091696837, -64.15931121805825, -64.66413151581865, -65.16889352423487, -65.67358895729222, -66.17820952897598, -66.68274695327148, -67.18719294416401, -67.69153921563887, -68.19577748168139, -68.69989945627682, -69.20389685341053, -69.53980106644636, -69.53980106644636, -70.03904068922449, -70.53824534388608, -71.03741850393202, -71.53656364286319, -72.03568423418045, -72.53478375138471, -73.03386566797683, -73.53293345745773, -74.03199059332825, -74.5310405490893, -75.03008679824175, -75.52913281428651, -76.02818207072443, -76.5272380410564, -77.02630419878331, -77.52538401740605, -78.02448097042549, -78.52359853134253, -79.02274017365804, -79.52190937087288, -80.02110959648799, -80.5203443240042, -81.01961702692243, -81.51893117874353, -82.01829025296841, -82.51769772309794, -83.01715706263303, -83.51667174507452, -84.01624524392331, -84.5158810326803, -85.01558258484634, -85.51535337392235, -86.0151968734092, -86.51398695208124, -86.51398695208124, -87.01378481453521, -87.51359137792667, -88.01340613342705, -88.51322857220782, -89.01305818544041, -89.51289446429632, -90.01273689994701, -90.51258498356393, -91.01243820631852, -91.5122960593823, -92.01215803392664, -92.51202362112309, -93.01189231214308, -93.51176359815807, -94.01163697033948, -94.51151191985885, -95.01138793788758, -95.51126451559716, -96.01114114415904, -96.51101731474469, -97.01089251852558, -97.51076624667314, -98.01063799035886, -98.5105072407542, -99.01037348903058, -99.51023622635952, -100.01009494391245, -100.50994913286084, -101.00979828437613, -101.50964188962982, -102.00947943979334, -102.50931042603817, -103.00913433953575, -103.50895067145754, -104.00875891297504, -104.50855855525968, -105.00834908948293, -105.50813000681626, -106.0079007984311, -106.50766095549893, -107.00740996919122, -107.50714733067944, -108.00687253113502, -108.50658506172944, -109.00628441363415, -109.50505830995377]
  out "x 7":dbl[](array[numeric])=[0.0, -0.062285707493046516, -0.2310475110116812]
  out "y 7":dbl[](array[numeric])=[0.0, 3.113870125529085, 5.994064450521981]
  out "y 8":dbl[](array[numeric])=[-40.25486400827094, -40.04085960963455, -39.821235299880705, -39.59593792545196, -39.364914332790825, -39.12811136833988, -38.88547587854164, -38.636954709838655, -38.382494708673484, -38.12204272148863, -37.85554559472668, -37.58295017483014, -37.30420330824157, -37.0192518414035, -36.728042620758494, -36.43052249274907, -36.126638303817785, -35.81633690040717, -35.49956512895978, -35.176269835918156, -34.846397867724825, -34.50989607082233, -34.166711291653236, -33.81679037666006, -33.460080172285366, -33.09652752497168, -32.72607928116154, -32.3486822872975, -31.96428338982209, -31.57282943517787, -31.17426726980736, -30.768543740153135, -30.355605692657697, -30.338651341222633, -30.338651341222633, -29.95729378436619, -29.572397676750224, -29.183911226613308, -28.791782642194068, -28.395960131731087, -27.996391903462964, -27.593026165628288, -27.185811126465662, -26.774694994213668, -26.359625977110902, -25.940552283395995, -25.5174221213075, -25.090183699084033, -24.658785224964184, -24.22317490718656, -23.783300953989748, -23.33911157361234, -22.89055497429293, -22.43757936427013, -21.980132951782515, -21.5181639450687, -21.05162055236726, -20.58045098191681, -20.10460344195595, -19.62402614072324, -19.138667286457324, -18.648475087396758, -18.153397751780158, -17.653383487846114, -17.14838050383323, -16.6383370079801, -16.123201208525305, -15.602921313707439, -15.077445531765132, -14.546722070936944, -14.010699139461483, -13.469324945577348, -12.922547697523145, -12.370315603537431, -11.812576871858855, -11.249279710725965, -10.68037232837739, -10.105802933051706, -9.52551973298753, -8.939470936423437, -8.347604751598034, -8.312579060465806, -8.312579060465806, -7.815979397588906, -7.318560473773825, -6.820356240811432, -6.321400650492564, -5.8217276546080905, -5.321371204948849, -4.820365253305692, -4.318743751469474, -3.816540651231034, -3.313789904381253, -2.8105254627109564, -2.3067812780109964, -1.8025913020722415, -1.2979894866855162, -0.7930097836417018, -0.2876861447316371, 0.2179474782538381, 0.7238571335238572, 1.2300088692875666, 1.7363687337541345, 2.2429027751326935, 2.7495770416323975, 3.2563575814623866, 3.763210442831828, 4.270101673949855, 4.776997323025622, 5.283863438268267, 5.79066606788696, 6.297371260090832, 6.803945063089038, 7.310353525090725, 7.816562694305046, 8.322538618941149, 8.82824734720817, 9.333654927315276, 9.532792066869051, 9.532792066869058, 10.032676667529001, 10.532532309358876, 11.032359899557544, 11.53216034532386, 12.03193455385667, 12.53168343235485, 13.03140788801724, 13.531108828042706, 14.030787159630101, 14.530443789978285, 15.030079626286113, 15.529695575752449, 16.029292545576137, 16.52887144295605, 17.028433175091028, 17.527978649179936, 18.02750877242164, 18.527024452014977, 19.026526595158828, 19.526016109052026, 20.025493900893448, 20.52496087788194, 21.02441794721636, 21.523866016095567, 22.023305991718424, 22.522738781283774, 23.022165291990486, 23.521586431037413, 24.021003105623414, 24.520416222947343, 25.01982669020806, 25.51923541460442, 26.018643303335274, 26.518051263599492, 27.017460202595917, 27.51687102752342, 28.016284645580857, 28.515701963967068, 29.01512388988093, 29.51455133052128, 30.013985193087, 30.513426384776935, 31.012875812789932, 31.512334384324856, 32.01180300658057, 32.511282586755925, 33.01077403204978, 33.51027824966099, 34.00979614678842, 34.15163746485512, 34.15163746485511, 34.65085156194158, 35.150114036225105, 35.649423358614406, 36.148778000018126, 36.64817643134495, 37.14761712350358, 37.64709854740265, 38.14661917395086, 38.64617747405689, 39.14577191862942, 39.6454009785771, 40.14506312480863, 40.644756828232666, 41.14448055975791, 41.644232790293024, 42.14401199074667, 42.643816632027544, 43.14364518504432, 43.64349612070567, 44.14336790992027, 44.6432590235968, 45.14316793264393, 45.64309310797034, 46.143033020484694, 46.64298614109569, 47.14295094071199, 47.64292589024228, 48.14290946059522, 48.64290012267951, 49.142896347403784, 49.64289660567677, 50.142899368407114, 50.64290310650349, 51.14290629087459, 51.64290739242908, 52.14290488207564, 52.64289723072293, 53.142882909279656, 53.642860388654476, 54.14282813975608, 54.64278463349311, 55.14272834077427, 55.64265773250823, 56.14257127960367, 56.642467452969264, 57.142344723513695, 57.642201562145615, 58.14203643977374, 58.6418478273067, 59.141634195653204, 59.641394015721914, 60.1411257584215, 60.64082789466066, 61.14049889534806, 61.64013723139237, 62.139741373702265, 62.63930979318643, 63.138840960753534, 63.63833334731226, 64.13778542377129, 64.63719566103929, 65.1365625300249, 65.63588450163687, 66.13516004678382, 66.62661681170006, 66.62661681170006, 67.12576345342403, 67.62478981859165, 68.1236869902195, 68.62244605132406, 69.12105808492187, 69.61951417402948, 70.11780540166339, 70.61592285084015, 71.11385760457627, 71.61160074588827, 72.10914335779272, 72.6064765233061, 73.10359132544497, 73.60047884722584, 74.09713017166524, 74.59353638177971, 75.08968856058576, 75.58557779109994, 76.08119515633875, 76.57653173931875, 77.07157862305642, 77.56632689056836, 78.060767624871, 78.55489190898098, 79.04869082591473, 79.54215545868882, 80.03527689031979, 80.52804620382416, 81.02045448221844, 81.51249280851917, 82.00415226574289, 82.49542393690609, 82.98629890502534, 83.47676825311716, 83.96682306419804, 84.45645442128455, 84.9456534073932, 85.43441110554052, 85.92271859874306, 86.4105669700173, 86.89794730237979, 87.17622393756727, 87.17622393756727, 87.62090998324233, 88.06278904034333, 88.5018353078985, 88.93802298493607, 89.37132627048422, 89.80171936357122, 90.22917646322526, 90.65367176847454, 91.07517947834734, 91.49367379187183, 91.90912890807624, 92.3215190259888, 92.73081834463773, 93.13700106305124, 93.54004138025758, 93.93991349528491, 94.3365916071615, 94.73004991491554, 95.12026261757528, 95.50720391416891, 95.89084800372467, 96.27116908527078, 96.64814135783546, 97.02173902044692, 97.39193627213336, 97.75870731192305, 98.12202633884417, 98.48186755192496, 98.83820515019363, 99.19101333267841, 99.54026629840749, 99.88593824640913, 99.89953643323281, 99.89953643323281, 100.21054094201504, 100.51734678566943, 100.81989169992012, 101.11811342049135, 101.41194968310735, 101.70133822349231, 101.98621677737043, 102.26652308046596, 102.54219486850307, 102.81316987720602, 103.07938584229896, 103.34078049950615, 103.59729158455178, 103.84885683316006, 104.09541398105519, 104.33690076396141, 104.5732549176029, 104.80441417770389, 105.0303162799886, 105.2508989601812, 105.46609995400595, 105.67585699718703, 105.88010782544866, 106.07879017451506, 106.27184178011042, 106.45920037795898, 106.64080370378494, 106.81658949331246, 106.98649548226584, 107.15045940636924, 107.30841900134685, 107.46031200292295, 107.60607614682168, 107.74564916876727, 107.87896880448396, 108.00597278969595, 108.12659886012742, 108.24078475150262, 108.34846819954572, 108.44958693998096, 108.54407870853257, 108.63188124092471, 108.71293227288164, 108.78716954012754, 108.85453077838663, 108.91495372338314, 108.96837611084122, 108.97747618937277, 108.97747618937277, 109.0156550246946, 109.04983247580746, 109.08011123358501, 109.10659398890081, 109.12938343262847, 109.14858225564154, 109.16429314881364, 109.17661880301837, 109.18566190912927, 109.19152515801999, 109.19431124056405, 109.19412284763511, 109.1910626701067, 109.18523339885247, 109.17673772474595, 109.16567833866077, 109.15215793147051, 109.13627919404871, 109.11814481726906, 109.09785749200506, 109.07551990913035, 109.05123475951848, 109.02510473404305, 108.99723252357771, 108.96772081899594, 108.93667231117144, 108.90418969097772, 108.87037564928839, 108.83533287697705, 108.79916406491728, 108.7619719039827, 108.72385908504685, 108.68492829898334, 108.64528223666576, 108.60502358896771, 108.56425504676278, 108.52307930092454, 108.48159904232658, 108.4399169618425, 108.39813575034592, 108.35635809871036, 108.31468669780945, 108.27322423851678, 108.23207341170594, 108.19133690825049, 108.15111741902408, 108.11151763490025, 108.07264024675257, 108.03458794545469, 107.99746342188017, 107.96136936690259, 107.92640847139555, 107.89268342623265, 107.86029692228745, 107.82935165043357, 107.79995030154457, 107.78125898031978, 107.78125898031978, 107.75369240153198, 107.72548456275034, 107.69669916249154, 107.66739989927227, 107.63765047160923, 107.60751457801909, 107.57705591701853, 107.54633818712422, 107.51542508685286, 107.48438031472112, 107.45326756924571, 107.42215054894329, 107.39109295233057, 107.36015847792419, 107.32941082424084, 107.29891368979723, 107.26873077311004, 107.23892577269594, 107.2095623870716, 107.18070431475374, 107.15241525425903, 107.12475890410411, 107.09779896280573, 107.07159912888052, 107.04622310084521, 107.02173457721644, 106.9981972565109, 106.97567483724531, 106.95423101793631, 106.9339294971006, 106.91483397325487, 106.89700814491579, 106.88051571060006, 106.86545285263342, 106.86545285263342, 106.85123591176482, 106.8373215059327, 106.82369194296759, 106.81032953069995, 106.79721657696027, 106.78433538957903, 106.7716682763867, 106.75919754521381, 106.74690550389077, 106.73477446024813, 106.72278672211637, 106.71092459732593, 106.69917039370733, 106.68750641909104, 106.67591498130754, 106.66437838818732, 106.65287894756085, 106.64139896725864, 106.62992075511116, 106.61842661894889, 106.60689886660232, 106.59531980590192, 106.5836717446782, 106.57193699076163, 106.56009785198269, 106.54813663617186, 106.53603565115962, 106.52377720477648, 106.51134360485288, 106.49871715921937, 106.4858801757064, 106.47281496214443, 106.45950382636393, 106.44592907619545, 106.43207301946944, 106.41791796401637, 106.40344621766674, 106.38864008825105, 106.37348188359975, 106.35795391154335, 106.34203847991229, 106.32571789653713, 106.30897446924827, 106.29179050587625, 106.27414831425155, 106.2560637066309]
  out "x 8":dbl[](array[numeric])=[-22.968902627554595, -22.51700484334325, -22.067726202847595, -21.62109147813308, -21.177125441265126, -20.735852864309198, -20.297298519330727, -19.86148717839516, -19.42844361356793, -18.998192596914485, -18.57075890050028, -18.146167296390736, -17.724442556651315, -17.305609453347444, -16.889692758544577, -16.476717244308148, -16.0667076827036, -15.659688845796383, -15.255685505651932, -14.854722434335699, -14.456824403913117, -14.062016186449632, -13.67032255401068, -13.28176827866172, -12.896378132468183, -12.514176887495505, -12.135189315809143, -11.759440189474532, -11.38695428055711, -11.017756361122329, -10.651871203235629, -10.289323578962446, -9.930138260368233, -9.915595940630572, -9.915595940630572, -9.592217431479307, -9.27296664733781, -8.957904003376973, -8.64708991476769, -8.340584796680856, -8.038449064287356, -7.740743132758091, -7.447527417263952, -7.158862332975826, -6.874808295064605, -6.595425718701188, -6.320775019056462, -6.05091661130132, -5.7859109106066535, -5.525818332143363, -5.270699291082332, -5.02061420259445, -4.775623481850621, -4.535787544021732, -4.301166804278667, -4.071821677792334, -3.8478125797336116, -3.6291999252734, -3.4160441295825903, -3.2084056078320766, -3.0063447751927437, -2.809922046835485, -2.619197837931207, -2.4342325636507813, -2.255086639165114, -2.0818204796450988, -1.9144945002616136, -1.7531691161855663, -1.597904742587841, -1.4487617946393383, -1.3058006875109367, -1.1690818363735358, -1.0386656563980352, -0.9146125627553217, -0.796982970616279, -0.6858372951518088, -0.581235951532802, -0.4832393549301528, -0.3919079205147527, -0.30730206345748806, -0.22948219892925836, -0.22511372738602808, -0.22511372738602808, -0.16680067513880384, -0.11507613036628858, -0.06966705231019729, -0.03030040021222455, 0.0032968666859287954, 0.03139778914256819, 0.05427540791599236, 0.07220276376450722, 0.08545289744639678, 0.09429884971998208, 0.09901366134354672, 0.09987037307539658, 0.09714202567383796, 0.0911016598971616, 0.08202231650367428, 0.0701770362516814, 0.055838859899467026, 0.0392808282053517, 0.020775981927619973, 0.0005973618245841139, -0.020981991345463767, -0.043689036824225154, -0.06725073385338684, -0.09139404167465787, -0.11584591952973904, -0.14033332666033183, -0.164583222308123, -0.18832256571482164, -0.21127831612212852, -0.233177432771738, -0.25374687490535136, -0.27271360176467, -0.28980457259138814, -0.30474674662721396, -0.31726708311384183, -0.32147712013105156, -0.3214771201310518, -0.3322441522303675, -0.3444544578596952, -0.3580628233106866, -0.37302403487498664, -0.38929287884424707, -0.4068241415101202, -0.4255726091642576, -0.44549306809831846, -0.4665403046039335, -0.4886691049727688, -0.5118342554964762, -0.5359905424667011, -0.5610927521750875, -0.5870956709133022, -0.6139540849729826, -0.6416227806457879, -0.670056544223363, -0.6992101619973595, -0.72903842025943, -0.7594961053012258, -0.7905380034143993, -0.8221189008906022, -0.8541935840214723, -0.8867168390986828, -0.9196434524138646, -0.9529282102586762, -0.9865258989247632, -1.0203913047037911, -1.0544792138873982, -1.088744412767236, -1.1231416876349567, -1.1576258247822122, -1.192151610500654, -1.2266738310819347, -1.261147272817699, -1.2955267219995985, -1.329766964919293, -1.3638227878684193, -1.3976489771386371, -1.4312003190215978, -1.4644315998089543, -1.4972976057923506, -1.5297531232634387, -1.5617529385138709, -1.593251837835299, -1.6242046075193748, -1.6545660338577437, -1.684290903142064, -1.713334001663981, -1.7214502693093892, -1.721450269309389, -1.7494765704663608, -1.7766543195019637, -1.803010337186423, -1.8285714442899548, -1.8533644615827702, -1.8774162098350855, -1.9007535098171258, -1.9234031822991002, -1.9453920480512341, -1.966746927843737, -1.9874946424468334, -2.00766201263074, -2.027275859165667, -2.046363002821832, -2.0649502643694664, -2.083064464578773, -2.1007324242199688, -2.1179809640632783, -2.1348369048789184, -2.1513270674370997, -2.1674782725080464, -2.183317340861975, -2.198871093269103, -2.2141663504996414, -2.229229933323813, -2.244088662511829, -2.2587693588339204, -2.27329884306029, -2.2877039359611624, -2.3020114583067546, -2.316248230867277, -2.3304410744129536, -2.3446168097140014, -2.358802257540638, -2.3730242386630804, -2.387309573851546, -2.401685083876244, -2.4161775895074067, -2.430813911515237, -2.445620870669959, -2.46062528774179, -2.4758539835009468, -2.491333778717647, -2.5070914941621076, -2.523153950604546, -2.539547968815179, -2.556300369564224, -2.573437973621899, -2.5909876017584192, -2.6089760747440036, -2.6274302133488687, -2.646376838343232, -2.66584277049731, -2.68585483058132, -2.7064398393654807, -2.7276246176200143, -2.749435986115125, -2.7719007656210435, -2.7950457769079735, -2.818897840746146, -2.843483777905771, -2.8688304091570727, -2.8949645552702545, -2.921913037015548, -2.9492635082994942, -2.9492635082994942, -2.978480917327609, -3.0098270674333767, -3.043459777809386, -3.079536867648219, -3.118216156142463, -3.1596554624846984, -3.204012605867507, -3.2514454054834765, -3.3021116805251873, -3.3561692501852223, -3.4137759336561606, -3.4750895501305976, -3.5402679188011072, -3.6094688588602786, -3.682850189500691, -3.760569729914927, -3.842785299295573, -3.929654716835212, -4.021335801726423, -4.117986373161795, -4.219764250333915, -4.326827252435352, -4.439333198658707, -4.557439908196553, -4.6813052002414715, -4.811086893986051, -4.946942808622881, -5.089030763344532, -5.237508577343594, -5.392534069812648, -5.554265059944274, -5.722859366931069, -5.898474809965605, -6.081269208240471, -6.27140038094824, -6.469026147281509, -6.674304326432857, -6.88739273759486, -7.10844919996011, -7.33763153272119, -7.5750975550706805, -7.714565866361133, -7.714565866361133, -7.943178762901428, -8.177335605648189, -8.417087352842183, -8.6624849627242, -8.913579393535008, -9.170421603515402, -9.433062550906158, -9.701553193948051, -9.975944490881862, -10.256287399948372, -10.542632879388364, -10.835031887442614, -11.133535382351901, -11.438194322357017, -11.74905966569872, -12.06618237061781, -12.389613395355056, -12.719403698151243, -13.055604237247149, -13.398265970883559, -13.747439857301249, -14.10317685474099, -14.465527921443577, -14.83454401564979, -15.210276095600387, -15.592775119536174, -15.982092045697918, -16.378277832326408, -16.78138343766241, -17.19145981994672, -17.608557937420102, -18.032728748323343, -18.0496518526286, -18.0496518526286, -18.441165968034287, -18.83605201755941, -19.234360005438532, -19.636139935906236, -20.041441813197096, -20.450315641545686, -20.862811425186578, -21.278979168354343, -21.698868875283566, -22.122530550208822, -22.550014197364675, -22.98136982098571, -23.41664742530649, -23.8558970145616, -24.29916859298561, -24.746512164813097, -25.197977734278638, -25.6536153056168, -26.113474883062164, -26.5776064708493, -27.046060073212793, -27.5188856943872, -27.996133338607113, -28.4778530101071, -28.96409471312173, -29.454908451885586, -29.950344230633245, -30.450452053599268, -30.95528192501824, -31.46488384912474, -31.979307830153324, -32.49860387233859, -33.0228219799151, -33.552012157117424, -34.08622440818015, -34.625508737337846, -35.16991514882508, -35.719493646876444, -36.2742942357265, -36.83436691960981, -37.39976170276098, -37.97052858941455, -38.54671758380513, -39.12837869016727, -39.71556191273555, -40.308317255744555, -40.90669472342885, -41.01788165020217, -41.01788165020217, -41.516426075908484, -42.01529336894664, -42.514475243301945, -43.01396341295969, -43.51374959190518, -44.013825494123736, -44.514182833600636, -45.01481332432121, -45.515708680270734, -46.01686061543453, -46.51826084379791, -47.019901079346155, -47.521773036064594, -48.0238684279385, -48.526178968953204, -49.02869637309399, -49.53141235434619, -50.03431862669508, -50.53740690412599, -51.04066890062418, -51.54409633017501, -52.04768090676373, -52.55141434437569, -53.055288356996165, -53.55929465861046, -54.0634249632039, -54.56767098476177, -55.072024437269384, -55.576477034712035, -56.08102049107504, -56.58564652034369, -57.090346836503294, -57.59511315353915, -58.09993718543659, -58.60481064618088, -59.109725249757346, -59.61467271015128, -60.119644741348004, -60.62463305733281, -61.129629372090996, -61.63462539960787, -62.13961285386874, -62.64458344885892, -63.149528898563695, -63.65444091696837, -64.15931121805825, -64.66413151581865, -65.16889352423487, -65.67358895729222, -66.17820952897598, -66.68274695327148, -67.18719294416401, -67.69153921563887, -68.19577748168139, -68.69989945627682, -69.20389685341053, -69.53980106644636, -69.53980106644636, -70.03904068922449, -70.53824534388608, -71.03741850393202, -71.53656364286319, -72.03568423418045, -72.53478375138471, -73.03386566797683, -73.53293345745773, -74.03199059332825, -74.5310405490893, -75.03008679824175, -75.52913281428651, -76.02818207072443, -76.5272380410564, -77.02630419878331, -77.52538401740605, -78.02448097042549, -78.52359853134253, -79.02274017365804, -79.52190937087288, -80.02110959648799, -80.5203443240042, -81.01961702692243, -81.51893117874353, -82.01829025296841, -82.51769772309794, -83.01715706263303, -83.51667174507452, -84.01624524392331, -84.5158810326803, -85.01558258484634, -85.51535337392235, -86.0151968734092, -86.51398695208124, -86.51398695208124, -87.01378481453521, -87.51359137792667, -88.01340613342705, -88.51322857220782, -89.01305818544041, -89.51289446429632, -90.01273689994701, -90.51258498356393, -91.01243820631852, -91.5122960593823, -92.01215803392664, -92.51202362112309, -93.01189231214308, -93.51176359815807, -94.01163697033948, -94.51151191985885, -95.01138793788758, -95.51126451559716, -96.01114114415904, -96.51101731474469, -97.01089251852558, -97.51076624667314, -98.01063799035886, -98.5105072407542, -99.01037348903058, -99.51023622635952, -100.01009494391245, -100.50994913286084, -101.00979828437613, -101.50964188962982, -102.00947943979334, -102.50931042603817, -103.00913433953575, -103.50895067145754, -104.00875891297504, -104.50855855525968, -105.00834908948293, -105.50813000681626, -106.0079007984311, -106.50766095549893, -107.00740996919122, -107.50714733067944, -108.00687253113502, -108.50658506172944, -109.00628441363415, -109.50505830995377]
  out "y 3":dbl[](array[numeric])
  out "x 3":dbl[](array[numeric])
  out "y 2":dbl[](array[numeric])
  out "x 2":dbl[](array[numeric])
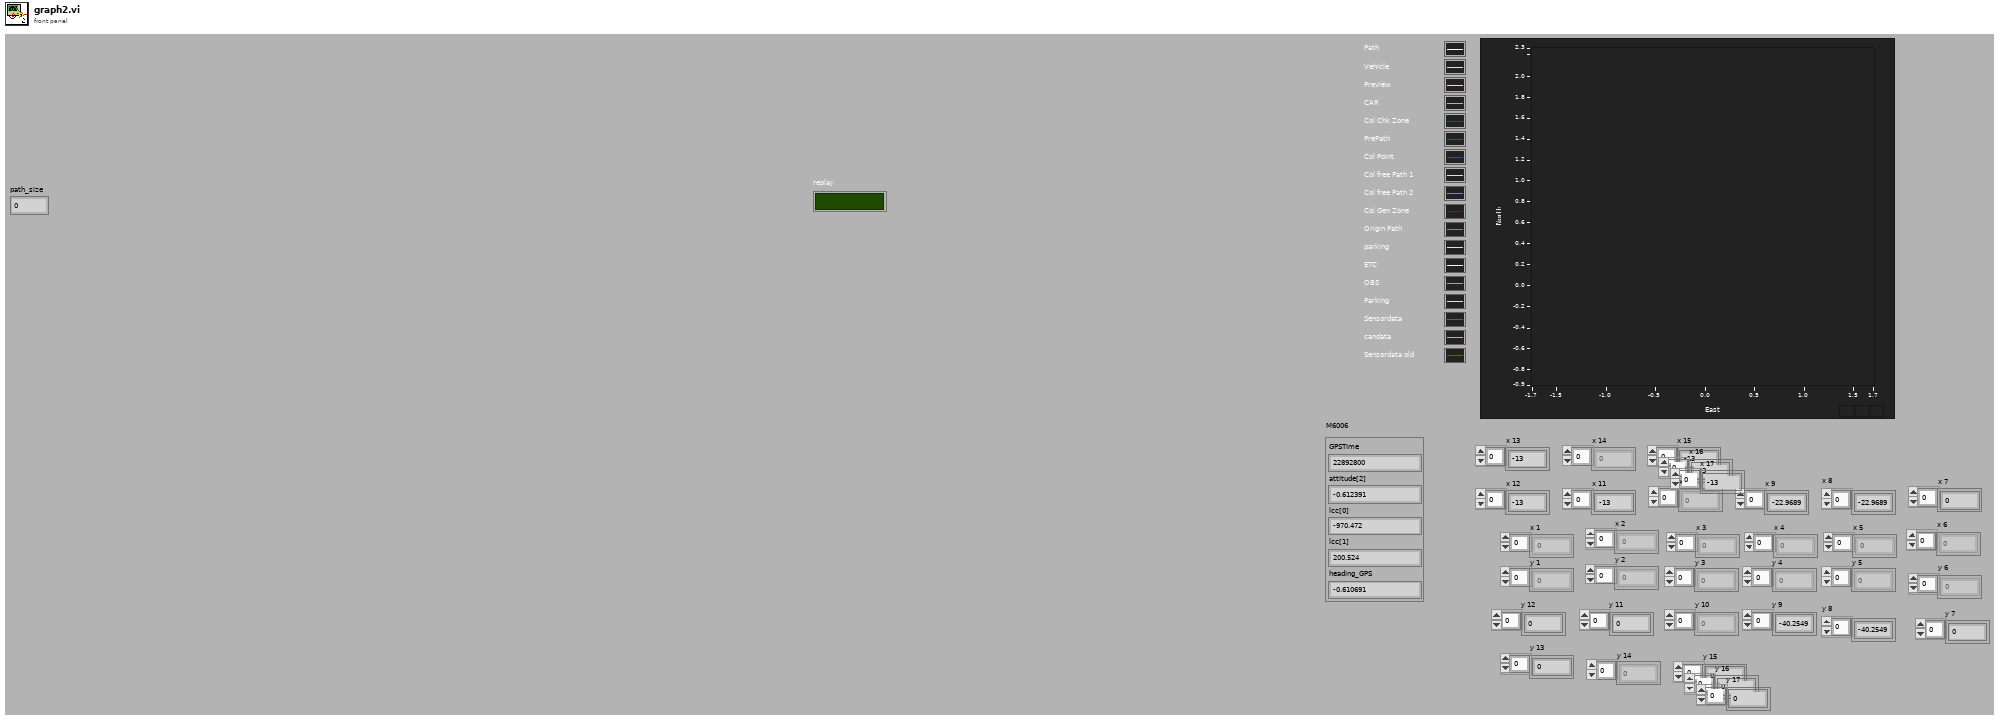
[diagram p1: front panel]
types:
  T1 = cluster{"GPSTime":dbl, "attitude[2]":sgl, "lcc[0]":sgl, "lcc[1]":sgl, "heading_GPS":sgl}
  T2 = typedef "NI_Matrix.lvlib/RealMatrix.ctl" = dbl[][]
  T3 = cluster{"GPSTime":dbl, "attitude[2]":dbl, "lcc[0]":dbl, "lcc[1]":dbl, "heading_GPS":dbl}
  T4 = cluster{"idx":i32, "x":dbl, "y":dbl, "h":dbl, "x_path":dbl}
  T5 = cluster{"idx":i32, "x":dbl, "y":dbl, "hp":dbl, "x_path":dbl}[]
  T6 = cluster{"hash":i64, "sys time":i64, "time":dbl, "x":dbl, "y":dbl, "h":dbl, "numSV":i32, "postype":i32, "lag":i32, "hordev":dbl, "lat":dbl, "lon":dbl, "hgt":dbl, "map_idx":i32}
  T7 = cluster{"hash":i64, "sys time":i64, "Auto":bool, "Run":bool, "Solenoid":bool, "T lim":bool, "brk_enc":u8, "B PWM":u16, "T PWM":u16, "ref_vel":dbl, "ref_bkr_enc":dbl, "ref_apv":dbl, "ref_steer":dbl}
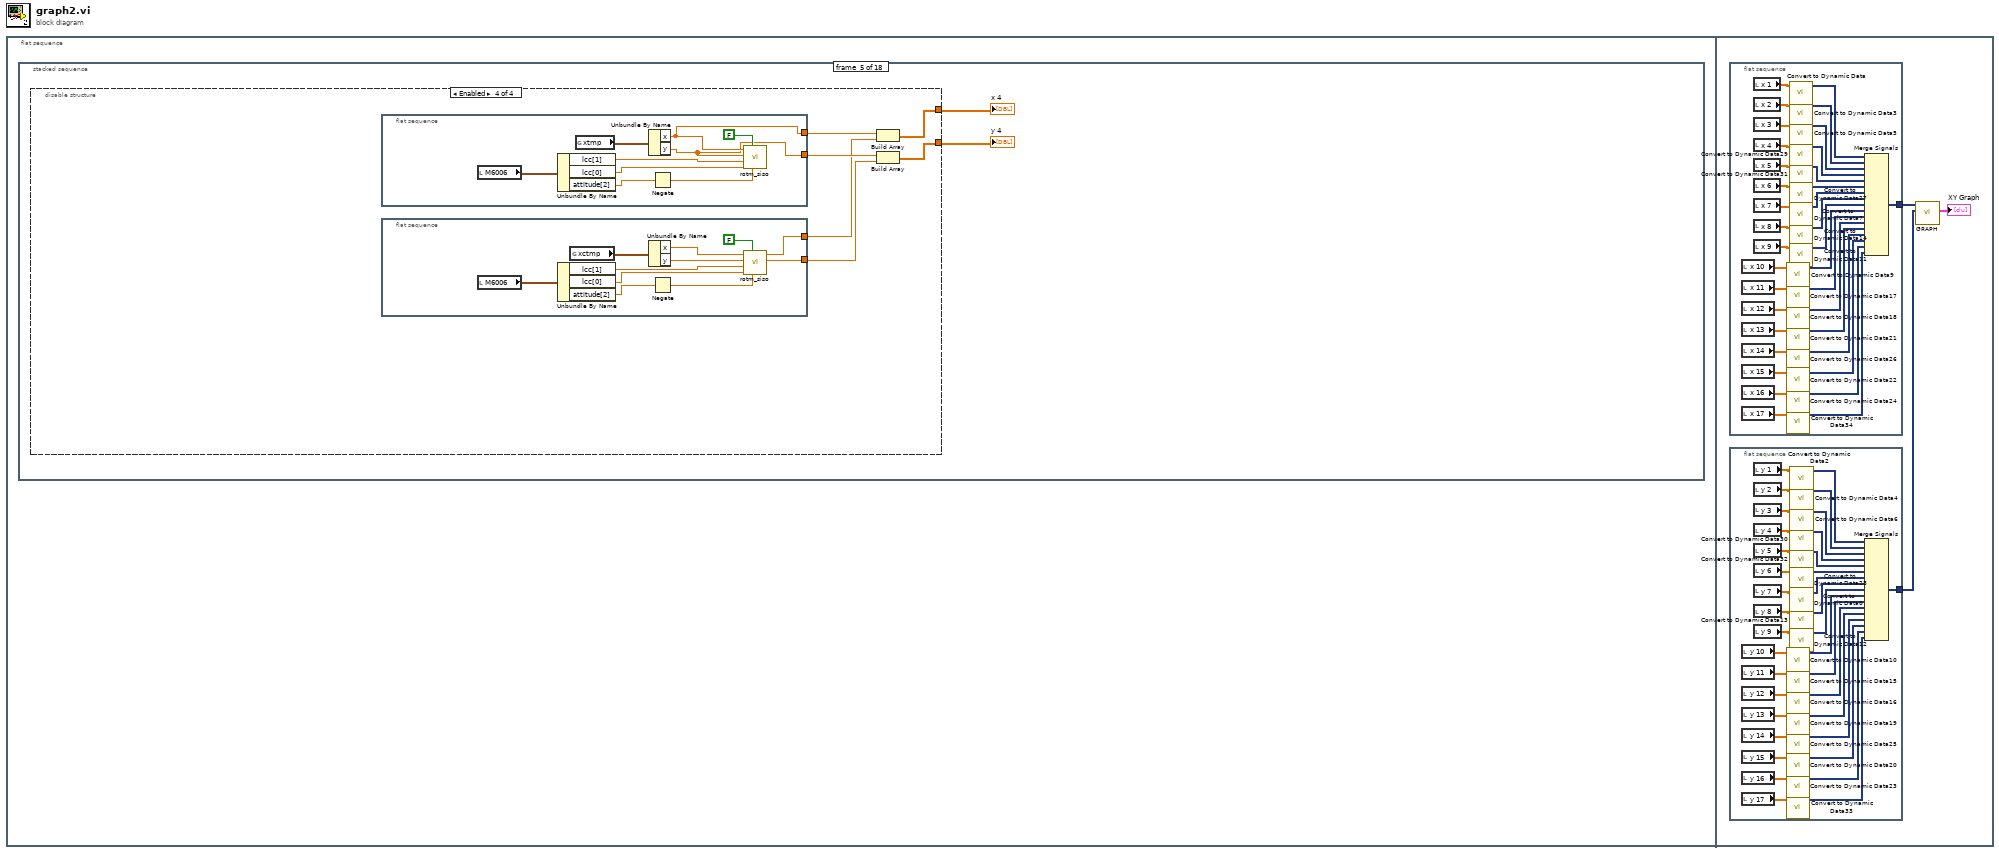
[diagram p0: block diagram]
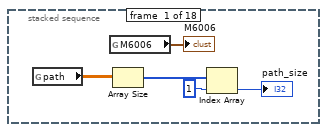
[diagram p2: hidden frame]
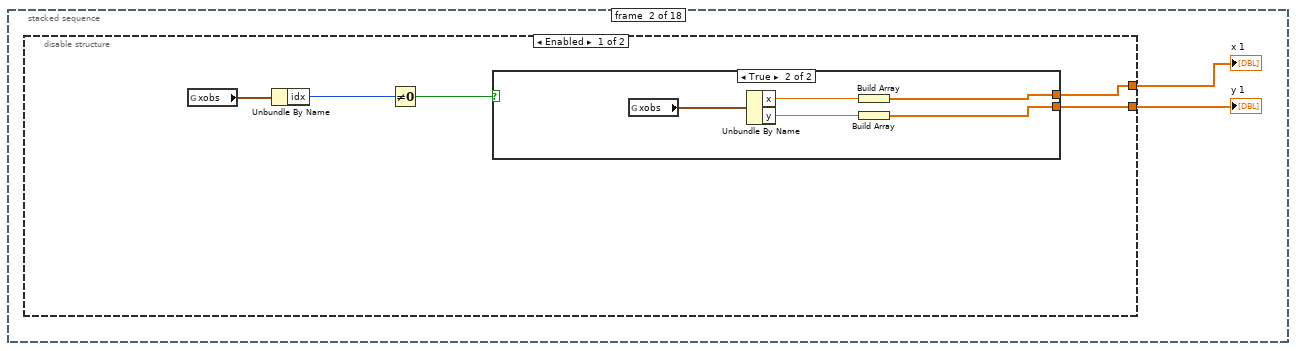
[diagram p3: hidden frame]
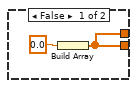
[diagram p4: hidden frame]
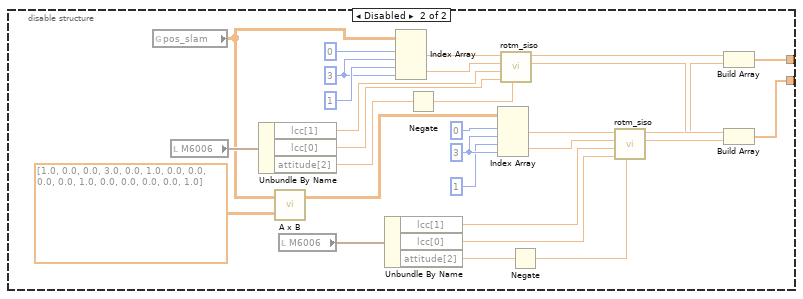
[diagram p5: hidden frame]
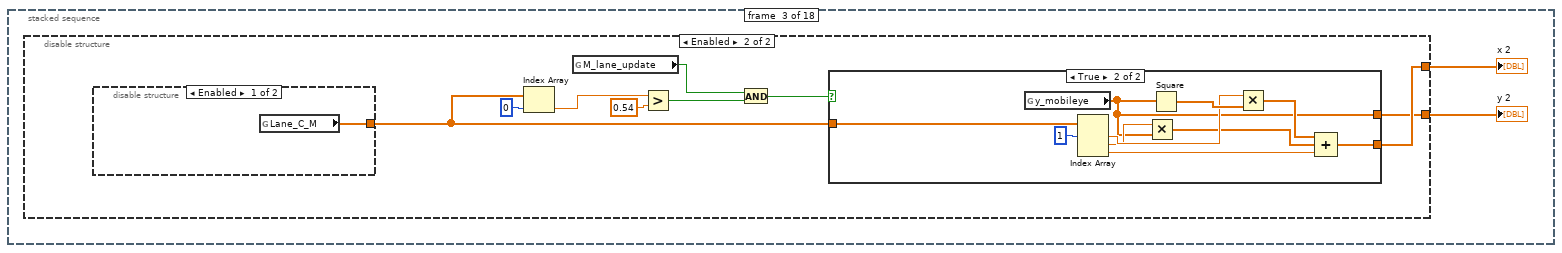
[diagram p6: hidden frame]
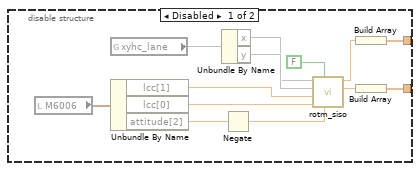
[diagram p7: hidden frame]
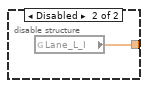
[diagram p8: hidden frame]
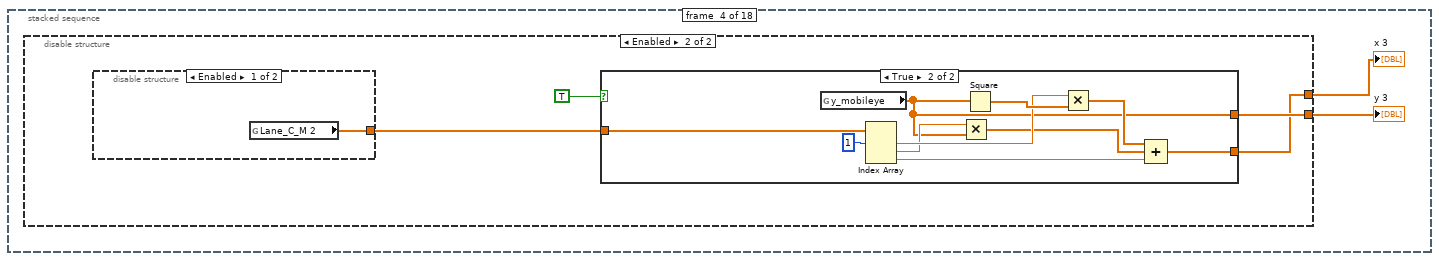
[diagram p10: hidden frame]
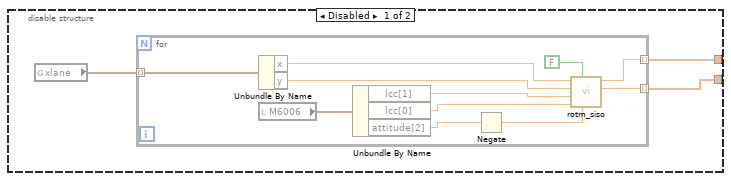
[diagram p11: hidden frame]
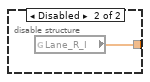
[diagram p12: hidden frame]
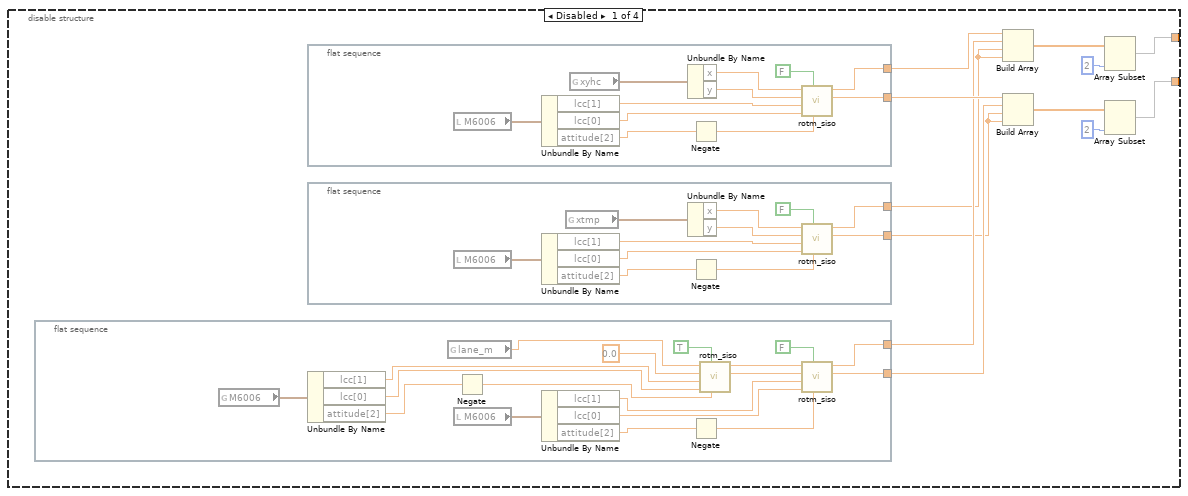
[diagram p14: hidden frame]
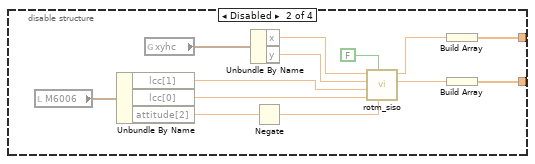
[diagram p15: hidden frame]
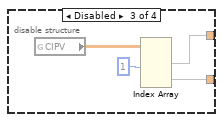
[diagram p16: hidden frame]
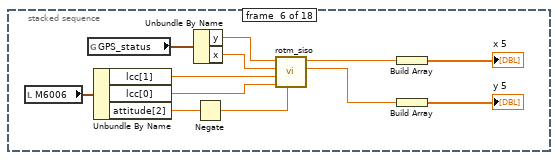
[diagram p17: hidden frame]
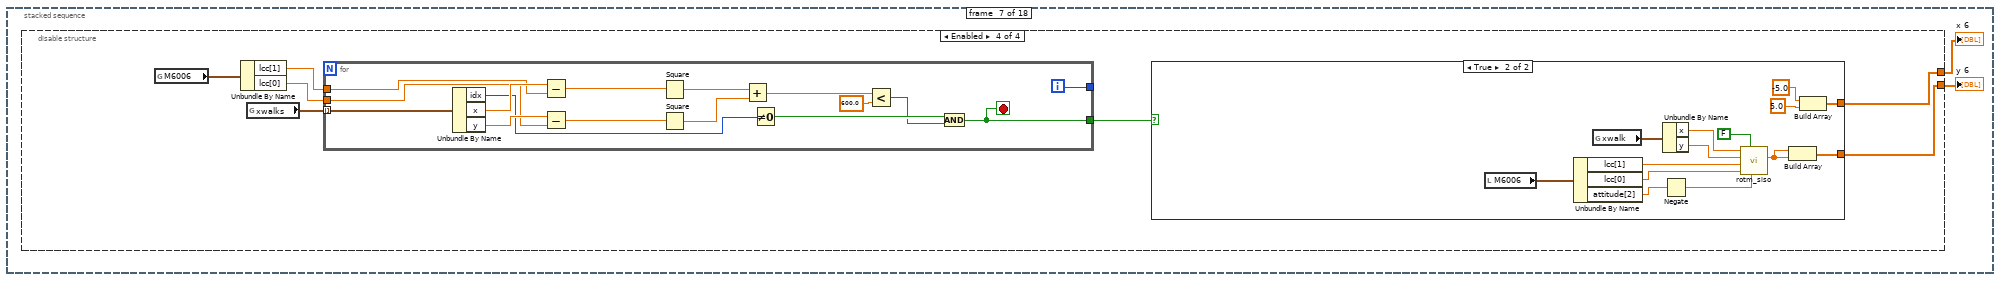
[diagram p18: hidden frame]
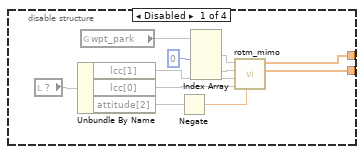
[diagram p19: hidden frame]
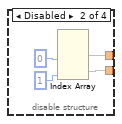
[diagram p20: hidden frame]
diagram:
  n1 = flat-sequence {
    frame #0 {
      n2 = stacked-sequence {
        frame #0 {
          n3 = global read "G_PATH.vi" "path"() -> (w2:dbl[][])
          n4 = global read "G_NAV.vi" "M6006"() -> (→"M6006":T3)
          n5 = Array Size(array=w2) -> (size(s)=w5:i32[])
          n6 = Index Array(array=w5, index=1) -> (element=→"path_size":i32)
        }
        frame #1 {
          n7 = disable-structure shown="Enabled" {
            disable-tunnel: [w9 w45] -> w7
            disable-tunnel: [w8 w44] -> w6
            frame Enabled {
              n8 = global read "G_VEH.vi" "xobs"() -> (w12:T4)
              n9 = Unbundle By Name(w12) -> ("idx"=w11:i32)
              n10 = Not Equal To 0?(x=w11) -> (x != 0?=w10:bool)
              n11 = case shown="True" w10 {
                tunnel: [w13 w19] -> w9
                tunnel: [w13 w18] -> w8
                frame False {
                  n12 = Build Array(0.0) -> (w13:dbl[])
                }
                frame True {
                  n13 = global read "G_VEH.vi" "xobs"() -> (w17:T4)
                  n14 = Unbundle By Name(w17) -> ("x"=w16:dbl, "y"=w15:dbl)
                  n15 = Build Array(w16) -> (w19:dbl[])
                  n16 = Build Array(w15) -> (w18:dbl[])
                }
              }
            }
            frame Disabled {
              w25 = 3 ("disabled index (col)")
              w46 = 3 ("disabled index (col)")
              n17 = global read "G_VEH.vi" "pos_slam"() -> (w33:T2)
              n18 = local read "M6006"() -> (w39:T1)
              n19 = Unbundle By Name(w39) -> ("lcc[1]"=w42:sgl, "lcc[0]"=w41:sgl, "attitude[2]"=w43:sgl)
              n20 = call-poly <vilib>:"A x B.vi"("B"=T2 [[1.0, 0.0, 0.0, 3.0], [0.0, 1.0, 0.0, 0.0], [0.0, 0.0, 1.0, 0.0], [0.0, 0.0, 0.0, 1.0]] ("pos_slam"), "A"=w33) -> ("A x B"=w22:T2)  [unwired: 1 out]
              n21 = local read "M6006"() -> (w30:T1)
              n22 = Unbundle By Name(w30) -> ("lcc[1]"=w27:sgl, "lcc[0]"=w28:sgl, "attitude[2]"=w26:sgl)
              n23 = Index Array(array=w33, index (row) #1=0 ("disabled index (row)"), index (col) #1=w46, index (row) #2=1 ("index (row)"), index (col) #2=w46) -> (element #1=w38:dbl, element #2=w37:dbl)
              n24 = Negate(x=w43) -> (-x=w40:sgl)
              n25 = Index Array(array=w22, index (row) #1=0 ("disabled index (row)"), index (col) #1=w25, index (row) #2=1 ("index (row)"), index (col) #2=w25) -> (element #1=w31:dbl, element #2=w32:dbl)
              n26 = call "rotm_siso.vi"("angle[rad]"=w40, "y0"=w41, "x0"=w42, "y"=w37, "x"=w38) -> ("y'"=w35:dbl, "x'"=w36:dbl)  [unwired: 5 in]
              n27 = Negate(x=w26) -> (-x=w29:sgl)
              n28 = call "rotm_siso.vi"("angle[rad]"=w29, "y0"=w28, "x0"=w27, "y"=w32, "x"=w31) -> ("y'"=w20:dbl, "x'"=w21:dbl)  [unwired: 5 in]
              n29 = Build Array(w36, w21) -> (w45:dbl[])
              n30 = Build Array(w35, w20) -> (w44:dbl[])
            }
          }
          "x 1" <- w7
          "y 1" <- w6
        }
        frame #2 {
          n31 = disable-structure shown="Enabled" {
            disable-tunnel: [w52 w72] -> w50
            disable-tunnel: [w51 w71] -> w49
            frame Disabled {
              n32 = local read "M6006"() -> (w55:T1)
              n33 = global read "G_VEH.vi" "xyhc_lane"() -> (w63)
              n34 = Unbundle By Name(w55) -> ("lcc[1]"=w59:sgl, "lcc[0]"=w60:sgl, "attitude[2]"=w56:sgl)
              n35 = Unbundle By Name(w63) -> ("x"=w57, "y"=w58)
              n36 = Negate(x=w56) -> (-x=w61:sgl)
              n37 = call "rotm_siso.vi"("angle[rad]"=w61, "reverse"=FALSE, "y0"=w60, "x0"=w59, "y"=w58, "x"=w57) -> ("y'"=w53:dbl, "x'"=w54:dbl)  [unwired: 4 in]
              n38 = Build Array(w54) -> (w52:dbl[])
              n39 = Build Array(w53) -> (w51:dbl[])
            }
            frame Enabled {
              n40 = disable-structure shown="Enabled" {
                disable-tunnel: [w73 w74] -> w70
                frame Enabled {
                  n41 = global read "G_SEN.vi" "Lane_C_M"() -> (w73:dbl[])
                }
                frame Disabled {
                  n42 = global read "G_SEN.vi" "Lane_L_I"() -> (w74:dbl[])
                }
              }
              n43 = Index Array(array=w70, index=0) -> (element=w67:dbl)
              n44 = global read "G_SEN.vi" "M_lane_update"() -> (w65:bool)
              n45 = Greater?(x=w67, y=0.54) -> (0:w64:bool)
              n46 = And(x=w65, y=w64) -> (x .and. y?=w69:bool)
              n47 = case shown="True" w69 {
                tunnel: w70 -> [_ w76]
                tunnel: [_ w77] -> w72
                tunnel: [_ w75] -> w71
                frame False {
                }
                frame True {
                  n48 = global read "G_SEN.vi" "y_mobileye"() -> (w75:dbl[])
                  n49 = Index Array(array=w76, index #1=1 ("index")) -> (element #1=w82:dbl, element #2=w81:dbl, element #3=w78:dbl)  [unwired: 2 in]
                  n50 = Multiply(x=w81, y=w75) -> (x*y=w79:dbl[])
                  n51 = Square(x=w75) -> (x^2=w83:dbl[])
                  n52 = Multiply(x=w82, y=w83) -> (x*y=w80:dbl[])
                  n53 = Compound Arithmetic op=ADD(w80, w79, w78) -> (w77:dbl[])
                }
              }
            }
          }
          "x 2" <- w50
          "y 2" <- w49
        }
        frame #3 {
          n54 = disable-structure shown="Enabled" {
            disable-tunnel: [w88 w103] -> w86
            disable-tunnel: [w87 w104] -> w85
            frame Disabled {
              n55 = global read "G_VEH.vi" "xlane"() -> (w89:T5)
              n56 = for {
                tunnel: w89 -> [w100] mode=indexing
                tunnel: [w91] -> w88 mode=indexing
                tunnel: [w90] -> w87 mode=indexing
                n57 = Unbundle By Name(w100) -> ("x"=w94:dbl, "y"=w95:dbl)
                n58 = local read "M6006"() -> (w92:T1)
                n59 = Unbundle By Name(w92) -> ("lcc[1]"=w96:sgl, "lcc[0]"=w97:sgl, "attitude[2]"=w93:sgl)
                n60 = Negate(x=w93) -> (-x=w98:sgl)
                n61 = call "rotm_siso.vi"("angle[rad]"=w98, "reverse"=FALSE, "y0"=w97, "x0"=w96, "y"=w95, "x"=w94) -> ("y'"=w90:dbl, "x'"=w91:dbl)  [unwired: 4 in]
              }
            }
            frame Enabled {
              n62 = disable-structure shown="Enabled" {
                disable-tunnel: [w105 w106] -> w102
                frame Enabled {
                  n63 = global read "G_SEN.vi" "Lane_C_M 2"() -> (w105:dbl[])
                }
                frame Disabled {
                  n64 = global read "G_SEN.vi" "Lane_R_I"() -> (w106:dbl[])
                }
              }
              n65 = case shown="True" TRUE {
                tunnel: w102 -> [_ w108]
                tunnel: [_ w109] -> w103
                tunnel: [_ w107] -> w104
                frame False {
                }
                frame True {
                  n66 = global read "G_SEN.vi" "y_mobileye"() -> (w107:dbl[])
                  n67 = Index Array(array=w108, index #1=1 ("index")) -> (element #1=w114:dbl, element #2=w113:dbl, element #3=w110:dbl)  [unwired: 2 in]
                  n68 = Multiply(x=w113, y=w107) -> (x*y=w111:dbl[])
                  n69 = Square(x=w107) -> (x^2=w115:dbl[])
                  n70 = Multiply(x=w114, y=w115) -> (x*y=w112:dbl[])
                  n71 = Compound Arithmetic op=ADD(w112, w111, w110) -> (w109:dbl[])
                }
              }
            }
          }
          "x 3" <- w86
          "y 3" <- w85
        }
        frame #4 {
          n72 = disable-structure shown="Enabled" {
            disable-tunnel: [w124 w172 w185 w192] -> w118
            disable-tunnel: [w121 w171 w184 w190] -> w117
            frame Disabled {
              n73 = flat-sequence {
                tunnel: [w143] -> w128
                tunnel: [w142] -> w127
                frame #0 {
                  n74 = global read "G_NAV.vi" "M6006"() -> (w159:T3)
                  n75 = Unbundle By Name(w159) -> ("lcc[1]"=w158:dbl, "lcc[0]"=w157:dbl, "attitude[2]"=w156:dbl)
                  n76 = global read "G_SEN.vi" "lane_m"() -> (w154:dbl)
                  n77 = local read "M6006"() -> (w151:T1)
                  n78 = Negate(x=w156) -> (-x=w155:dbl)
                  n79 = Unbundle By Name(w151) -> ("lcc[1]"=w149:sgl, "lcc[0]"=w148:sgl, "attitude[2]"=w150:sgl)
                  n80 = Negate(x=w150) -> (-x=w146:sgl)
                  n81 = call "rotm_siso.vi"("angle[rad]"=w155, "reverse"=TRUE, "y0"=w157, "x0"=w158, "y"=0.0, "x"=w154) -> ("y'"=w144:dbl, "x'"=w145:dbl)  [unwired: 4 in]
                  n82 = call "rotm_siso.vi"("angle[rad]"=w146, "reverse"=FALSE, "y0"=w148, "x0"=w149, "y"=w144, "x"=w145) -> ("y'"=w142:dbl, "x'"=w143:dbl)  [unwired: 4 in]
                }
              }
              n83 = flat-sequence {
                tunnel: [w162] -> w130
                tunnel: [w161] -> w129
                frame #0 {
                  n84 = local read "M6006"() -> (w163:T1)
                  n85 = Unbundle By Name(w163) -> ("lcc[1]"=w167:sgl, "lcc[0]"=w168:sgl, "attitude[2]"=w164:sgl)
                  n86 = global read "G_VEH.vi" "xyhc"() -> (w160:T4)
                  n87 = Unbundle By Name(w160) -> ("x"=w165:dbl, "y"=w166:dbl)
                  n88 = Negate(x=w164) -> (-x=w169:sgl)
                  n89 = call "rotm_siso.vi"("angle[rad]"=w169, "reverse"=FALSE, "y0"=w168, "x0"=w167, "y"=w166, "x"=w165) -> ("y'"=w161:dbl, "x'"=w162:dbl)  [unwired: 4 in]
                }
              }
              n90 = flat-sequence {
                tunnel: [w133] -> w120
                tunnel: [w132] -> w119
                frame #0 {
                  n91 = local read "M6006"() -> (w134:T1)
                  n92 = Unbundle By Name(w134) -> ("lcc[1]"=w138:sgl, "lcc[0]"=w139:sgl, "attitude[2]"=w135:sgl)
                  n93 = global read "G_VEH.vi" "xtmp"() -> (w131:T4)
                  n94 = Unbundle By Name(w131) -> ("x"=w136:dbl, "y"=w137:dbl)
                  n95 = Negate(x=w135) -> (-x=w140:sgl)
                  n96 = call "rotm_siso.vi"("angle[rad]"=w140, "reverse"=FALSE, "y0"=w139, "x0"=w138, "y"=w137, "x"=w136) -> ("y'"=w132:dbl, "x'"=w133:dbl)  [unwired: 4 in]
                }
              }
              n97 = Build Array(w130, w128, w120, w120) -> (w126:dbl[])
              n98 = Build Array(w129, w127, w119, w119) -> (w122:dbl[])
              n99 = Array Subset(array=w126, length=2) -> (w124:dbl[])  [unwired: 1 in]
              n100 = Array Subset(array=w122, length=2) -> (w121:dbl[])  [unwired: 1 in]
            }
            frame Disabled {
              n101 = local read "M6006"() -> (w175:T1)
              n102 = Unbundle By Name(w175) -> ("lcc[1]"=w179:sgl, "lcc[0]"=w180:sgl, "attitude[2]"=w176:sgl)
              n103 = global read "G_VEH.vi" "xyhc"() -> (w183:T4)
              n104 = Unbundle By Name(w183) -> ("x"=w177:dbl, "y"=w178:dbl)
              n105 = Negate(x=w176) -> (-x=w181:sgl)
              n106 = call "rotm_siso.vi"("angle[rad]"=w181, "reverse"=FALSE, "y0"=w180, "x0"=w179, "y"=w178, "x"=w177) -> ("y'"=w173:dbl, "x'"=w174:dbl)  [unwired: 4 in]
              n107 = Build Array(w174) -> (w172:dbl[])
              n108 = Build Array(w173) -> (w171:dbl[])
            }
            frame Disabled {
              n109 = global read "G_SEN.vi" "CIPV"() -> (w187:dbl[][])
              n110 = Index Array(array=w187, index (col) #1=1 ("disabled index (col)")) -> (element #1=w185:dbl[], element #2=w184:dbl[])  [unwired: 3 in]
            }
            frame Enabled {
              n111 = flat-sequence {
                tunnel: [w206] -> w193
                tunnel: [w205] -> w191
                frame #0 {
                  n112 = local read "M6006"() -> (w208:T1)
                  n113 = Unbundle By Name(w208) -> ("lcc[1]"=w210:sgl, "lcc[0]"=w211:sgl, "attitude[2]"=w209:sgl)
                  n114 = global read "G_VEH.vi" "xtmp"() -> (w207:T4)
                  n115 = Unbundle By Name(w207) -> ("x"=w206:dbl, "y"=w205:dbl)
                  n116 = Negate(x=w209) -> (-x=w212:sgl)
                  n117 = call "rotm_siso.vi"("angle[rad]"=w212, "reverse"=FALSE, "y0"=w211, "x0"=w210, "y"=w205, "x"=w206) -> ()  [unwired: 4 in, 2 out]
                }
              }
              n118 = flat-sequence {
                tunnel: [w196] -> w189
                tunnel: [w195] -> w188
                frame #0 {
                  n119 = local read "M6006"() -> (w197:T1)
                  n120 = Unbundle By Name(w197) -> ("lcc[1]"=w201:sgl, "lcc[0]"=w202:sgl, "attitude[2]"=w198:sgl)
                  n121 = global read "G_VEH.vi" "xctmp"() -> (w194:T4)
                  n122 = Unbundle By Name(w194) -> ("x"=w199:dbl, "y"=w200:dbl)
                  n123 = Negate(x=w198) -> (-x=w203:sgl)
                  n124 = call "rotm_siso.vi"("angle[rad]"=w203, "reverse"=FALSE, "y0"=w202, "x0"=w201, "y"=w200, "x"=w199) -> ("y'"=w195:dbl, "x'"=w196:dbl)  [unwired: 4 in]
                }
              }
              n125 = Build Array(w193, w189) -> (w192:dbl[])
              n126 = Build Array(w191, w188) -> (w190:dbl[])
            }
          }
          "x 4" <- w118
          "y 4" <- w117
        }
        frame #5 {
          n127 = local read "M6006"() -> (w221:T1)
          n128 = global read "G_NAV.vi" "GPS_status"() -> (w216:T6)
          n129 = Unbundle By Name(w221) -> ("lcc[1]"=w224:sgl, "lcc[0]"=w223:sgl, "attitude[2]"=w225:sgl)
          n130 = Unbundle By Name(w216) -> ("y"=w215:dbl, "x"=w214:dbl)
          n131 = Negate(x=w225) -> (-x=w222:sgl)
          n132 = call "rotm_siso.vi"("angle[rad]"=w222, "y0"=w223, "x0"=w224, "y"=w214, "x"=w215) -> ("y'"=w218:dbl, "x'"=w220:dbl)  [unwired: 5 in]
          n133 = Build Array(w220) -> (→"x 5":dbl[])
          n134 = Build Array(w218) -> (→"y 5":dbl[])
        }
        frame #6 {
          n135 = disable-structure shown="Enabled" {
            disable-tunnel: [w237 w239 w246 w253] -> w227
            disable-tunnel: [w236 w240 w245 w254] -> w226
            frame Disabled {
              n136 = local read item#-1() -> (w228)
              n137 = Unbundle By Name(w228) -> ("lcc[1]"=w231, "lcc[0]"=w230, "attitude[2]"=w232)
              n138 = global read "G_SEN.vi" "wpt_park"() -> (w233)
              n139 = Negate(x=w232) -> (-x=w229:dbl)
              n140 = Index Array(array=w233, index (col) #1=0 ("disabled index (col)")) -> (element #1=w234, element #2=w235)  [unwired: 3 in]
              n141 = call "rotm_mimo.vi"("angle[rad]"=w229, "y0"=w230, "x0"=w231, "y"=w235, "x"=w234) -> ("Y"=w237:dbl[], "X"=w236:dbl[])  [unwired: 3 in, 2 out]
            }
            frame Disabled {
              n142 = Index Array(index (col) #1=0 ("disabled index (col)"), index (col) #2=1 ("index (col)")) -> (element #1=w240, element #2=w239)  [unwired: 3 in]
            }
            frame Disabled {
              n143 = global read "G_SEN.vi" "crosswalk"() -> (w247:dbl)
              n144 = Build Array(-5.0 ("element"), 5.0 ("element")) -> (w245:dbl[])
              n145 = Build Array(w247, w247) -> (w246:dbl[])
            }
            frame Enabled {
              n146 = global read "G_NAV.vi" "M6006"() -> (w252:T3)
              n147 = Unbundle By Name(w252) -> ("lcc[1]"=w251:dbl, "lcc[0]"=w250:dbl)
              n148 = global read "G_VEH.vi" "xwalks"() -> (w249:T5)
              n149 = for {
                tunnel: w249 -> [w270] mode=indexing
                tunnel: w251 -> [w268]
                tunnel: w250 -> [w266]
                tunnel: [w255] -> w248
                tunnel: [w259] -> _
                i -> [w259]
                stop <- w255 stop-if-true
                n150 = Unbundle By Name(w270) -> ("idx"=w258:i32, "x"=w269:dbl, "y"=w267:dbl)
                n151 = Subtract(x=w269, y=w268) -> (x-y=w264:dbl)
                n152 = Subtract(x=w267, y=w266) -> (x-y=w265:dbl)
                n153 = Square(x=w264) -> (x^2=w263:dbl)
                n154 = Square(x=w265) -> (x^2=w262:dbl)
                n155 = Add(x=w263, y=w262) -> (x+y=w261:dbl)
                n156 = Not Equal To 0?(x=w258) -> (x != 0?=w257:bool)
                n157 = Less?(x=w261, y=600.0) -> (x < y?=w256:bool)
                n158 = And(x=w257, y=w256) -> (x .and. y?=w255:bool)
              }
              n159 = case shown="True" w248 {
                tunnel: [_ w287] -> w254
                tunnel: [_ w286] -> w253
                frame False {
                  n160 = global read "G_NAV.vi" "M6006"() -> (w274:T3)
                  n161 = Unbundle By Name(w274) -> ("lcc[1]"=w271:dbl, "lcc[0]"=w272:dbl, "attitude[2]"=w275:dbl)
                  n162 = Negate(x=w275) -> (-x=w273:dbl)
                  n163 = call "rotm_siso.vi"("angle[rad]"=w273, "reverse"=TRUE, "y0"=w272, "x0"=w271, "y"=90.0, "x"=0.0) -> ("y'"=w281:dbl, "x'"=w280:dbl)  [unwired: 4 in]
                  n164 = global read "G_VEH.vi" "xwalk"() -> (w279:T4)
                  n165 = Bundle By Name(cluster=w279, "x"=w280, "y"=w281) -> (w282:T4)
                  n166 = global write "G_VEH.vi" "xwalk"(w282) -> ()
                }
                frame True {
                  n167 = local read "M6006"() -> (w288:T1)
                  n168 = Unbundle By Name(w288) -> ("lcc[1]"=w292:sgl, "lcc[0]"=w293:sgl, "attitude[2]"=w289:sgl)
                  n169 = global read "G_VEH.vi" "xwalk"() -> (w296:T4)
                  n170 = Unbundle By Name(w296) -> ("x"=w290:dbl, "y"=w291:dbl)
                  n171 = Negate(x=w289) -> (-x=w294:sgl)
                  n172 = call "rotm_siso.vi"("angle[rad]"=w294, "reverse"=FALSE, "y0"=w293, "x0"=w292, "y"=w291, "x"=w290) -> ("y'"=w283:dbl)  [unwired: 4 in, 1 out]
                  n173 = Build Array(w283, w283) -> (w286:dbl[])
                  n174 = Build Array(-5.0 ("element"), 5.0 ("element")) -> (w287:dbl[])
                }
              }
            }
          }
          "x 6" <- w226
          "y 6" <- w227
        }
        frame #7 {
          n175 = disable-structure shown="Enabled" {
            disable-tunnel: [w318 w338 w348] -> w313
            frame Disabled {
              n176 = global read "G_VEH.vi" "Rpath"() -> (w318:dbl)
            }
            frame Enabled {
              n177 = global read "G_LCM.vi" "CON_T"() -> (w331:T7)
              n178 = global read "G_VEH.vi" "ratio_steer"() -> (w336:dbl)
              n179 = global read "G_VEH.vi" "ratio_steer"() -> (w342:dbl)
              n180 = Unbundle By Name(w331) -> ("ref_steer"=w330:dbl)
              n181 = global read "G_VEH.vi" "handle"() -> (w340:dbl)
              n182 = Divide(x=w330, y=w336) -> (x/y=w337:dbl)
              n183 = Divide(x=w340, y=w342) -> (x/y=w341:dbl)
              n184 = Multiply(x=w337, y=3.141592653589793) -> (x*y=w333:dbl)
              n185 = Multiply(x=w341, y=3.141592653589793) -> (x*y=w346:dbl)
              n186 = Divide(x=w333, y=180.0) -> (x/y=w335:dbl)
              n187 = Divide(x=w346, y=180.0) -> (x/y=w344:dbl)
              n188 = global read "G_VEH.vi" "C_Wheel base"() -> (w320:dbl)
              n189 = global read "G_VEH.vi" "C_Wheel base"() -> (w343:dbl)
              n190 = Tangent(1:w335) -> (0:w321:dbl)
              n191 = Tangent(1:w344) -> (0:w328:dbl)
              n192 = Divide(x=w320, y=w321) -> (x/y=w323:dbl)
              n193 = Divide(x=w343, y=w328) -> (x/y=w327:dbl)
              n194 = Not Equal To 0?(x=w321) -> (x != 0?=w322:bool)
              n195 = Not Equal To 0?(x=w328) -> (x != 0?=w329:bool)
              n196 = Select(t=w323, s=w322, f=9999999.0) -> (s? t:f=w319:dbl)
              n197 = Select(t=w327, s=w329, f=9999999.0) -> (s? t:f=w326:dbl)
              n198 = local read "replay"() -> (w339:bool)
              n199 = Select(t=w319, s=w339, f=w326) -> (s? t:f=w338:dbl)
            }
            frame Disabled {
              n200 = global read "G_PATH.vi" "RXY"() -> (w353:dbl[])
              n201 = Index Array(array=w353, index #1=0 ("index")) -> (element #1=w349:dbl, element #2=w352:dbl)  [unwired: 1 in]
              n202 = Sign(1:w352) -> (0:w351:dbl)
              n203 = Negate(x=w351) -> (-x=w350:dbl)
              n204 = Multiply(x=w349, y=w350) -> (x*y=w348:dbl)
            }
          }
          n205 = disable-structure shown="Enabled" {
            disable-tunnel: [w315 30.0] -> w299
            frame Disabled {
              n206 = global read "G_VEH.vi" "Preview dist"() -> (w314:dbl)
              n207 = Multiply(x=w314, y=1.5) -> (x*y=w315:dbl)
            }
            frame Enabled {
            }
          }
          n208 = Divide(x=w299, y=w313) -> (x/y=w306:dbl)
          n209 = Equal To 0?(x=w313) -> (x = 0?=w305:bool)
          n210 = Select(t=0.0, s=w305, f=w306) -> (s? t:f=w303:dbl)
          n211 = Absolute Value(x=w303) -> (abs(x)=w304:dbl)
          n212 = Sign(1:w303) -> (0:w301:dbl)
          n213 = call "array_new.vi"("end"=w304, "size"=0.04, "start"=0.0) -> ("Array"=w302:dbl[])  [unwired: 7 in, 1 out]
          n214 = Multiply(x=w302, y=w301) -> (x*y=w300:dbl[])
          n215 = Sine & Cosine(0:w300) -> (1:w308:dbl[], 2:w309:dbl[])
          n216 = Multiply(x=w313, y=w308) -> (x*y=→"y 7":dbl[])
          n217 = Multiply(x=w309, y=w313) -> (x*y=w312:dbl[])
          n218 = Subtract(x=w312, y=w313) -> (x-y=→"x 7":dbl[])
        }
        frame #8 {
          n219 = disable-structure shown="Enabled" {
            disable-tunnel: [w357 w378] -> w356
            disable-tunnel: [w358 w379] -> w355
            frame Enabled {
              n220 = global read "G_PATH.vi" "map_track_saved"() -> (w365:dbl[][])
              n221 = global read "G_PATH.vi" "map_track"() -> (w366:dbl[][])
              n222 = local read "M6006"() -> (w361:T1)
              n223 = Unbundle By Name(w361) -> ("lcc[1]"=w360:sgl, "lcc[0]"=w359:sgl, "attitude[2]"=w363:sgl)
              n224 = Select(t=w365, s="replay", f=w366) -> (s? t:f=w364:dbl[][])
              n225 = Negate(x=w363) -> (-x=w362:sgl)
              n226 = Index Array(array=w364, index (col) #1=0 ("disabled index (col)"), index (col) #2=1 ("disabled index (col)")) -> (element #1=w358:dbl[], element #2=w357:dbl[])  [unwired: 2 in]
              n227 = call "rotm_mimo.vi"("angle[rad]"=w362, "y0"=w359, "x0"=w360, "y"=w357, "x"=w358) -> ()  [unwired: 3 in, 4 out]
            }
            frame Disabled {
              n228 = global read "G_SEN.vi" "y_mobileye"() -> (w378:dbl[])
              n229 = global read "G_SEN.vi" "Lane_C_M"() -> (w377:dbl[])
              n230 = Square(x=w378) -> (x^2=w375:dbl[])
              n231 = Index Array(array=w377, index #1=1 ("index")) -> (element #1=w374:dbl, element #2=w373:dbl, element #3=w370:dbl)  [unwired: 2 in]
              n232 = Multiply(x=w374, y=w375) -> (x*y=w372:dbl[])
              n233 = Multiply(x=w373, y=w378) -> (x*y=w371:dbl[])
              n234 = Compound Arithmetic op=ADD(w372, w371, w370) -> (w379:dbl[])
            }
          }
          "x 8" <- w355
          "y 8" <- w356
        }
        frame #9 {
          n235 = disable-structure shown="Enabled" {
            disable-tunnel: [w389 w420] -> w381
            disable-tunnel: [w388 w419] -> w380
            frame Enabled {
              n236 = disable-structure shown="Enabled" {
                disable-tunnel: [w398 w412 _] -> w383
                disable-tunnel: [w397 w413 _] -> w382
                frame Disabled {
                  n237 = global read "G_VEH.vi" "xyhc_shift"() -> (w410)
                  n238 = Unbundle By Name(w410) -> ("x"=w396, "y"=w395, "h"=w407)
                  n239 = call "headingoperater.vi"("h1"=w407, "h2"=1.5707963267948966) -> ("h2-h1"=w401:dbl)  [unwired: 8 in, 1 out]
                  n240 = global read "G_VEH.vi" "xyhc_lane"() -> (w399)
                  n241 = Unbundle By Name(w399) -> ("x"=w408, "y"=w409)
                  n242 = Negate(x=w401) -> (-x=w400:dbl)
                  n243 = call "rotm_siso.vi"("angle[rad]"=w400, "y0"=w395, "x0"=w396, "y"=w409, "x"=w408) -> ("x'"=w411:dbl)  [unwired: 5 in, 1 out]
                  n244 = call "rotm_siso.vi"("angle[rad]"=w400, "reverse"=TRUE, "y0"=w395, "x0"=w396, "y"=0.0, "x"=w411) -> ("y'"=w403:dbl, "x'"=w404:dbl)  [unwired: 4 in]
                  n245 = Subtract(x=w404, y=w396) -> (x-y=w397:dbl)
                  n246 = Subtract(x=w403, y=w395) -> (x-y=w398:dbl)
                }
                frame Disabled {
                  n247 = global read "G_PATH.vi" "xt"() -> (w413:dbl)
                  n248 = global read "G_PATH.vi" "yt"() -> (w412:dbl)
                }
                frame Enabled {
                }
              }
              n249 = local read "M6006"() -> (w390:T1)
              n250 = Unbundle By Name(w390) -> ("lcc[1]"=w393:sgl, "lcc[0]"=w392:sgl, "attitude[2]"=w394:sgl)
              n251 = global read "G_PATH.vi" "x origin"() -> (w387:dbl[])
              n252 = global read "G_PATH.vi" "y origin"() -> (w386:dbl[])
              n253 = Add(x=w387, y=w382) -> (x+y=w385:dbl[])
              n254 = Add(x=w386, y=w383) -> (x+y=w384:dbl[])
              n255 = Negate(x=w394) -> (-x=w391:sgl)
              n256 = call "rotm_mimo.vi"("angle[rad]"=w391, "y0"=w392, "x0"=w393, "y"=w384, "x"=w385) -> ("Y"=w388:dbl[], "X"=w389:dbl[])  [unwired: 3 in, 2 out]
            }
            frame Disabled {
              n257 = global read "G_SEN.vi" "Lane_C_I"() -> (w417:dbl[])
              n258 = Index Array(array=w417, index=0) -> (element=w416:dbl)
              n259 = Greater Or Equal?(x=w416, y=0.0) -> (x >= y?=w414:bool)
              n260 = case shown="True" w414 {
                tunnel: w417 -> [_ w425]
                tunnel: [_ w435] -> w420
                tunnel: [_ w423] -> w419
                frame False {
                }
                frame True {
                  n261 = Index Array(array=w425, index=1) -> (element=w422:dbl)
                  n262 = Absolute Value(x=w422) -> (abs(x)=w421:dbl)
                  n263 = Multiply(x=w421, y=2.0) -> (x*y=w432:dbl)
                  n264 = Reciprocal(x=w432) -> (1/x=w431:dbl)
                  n265 = Multiply(x=0.5, y=w431) -> (x*y=w429:dbl)
                  n266 = Round To Nearest(number=w429) -> (nearest integer value=w428:dbl)
                  n267 = Max & Min(x=w428, y=150.0) -> (max(x,y)=w426:dbl)  [unwired: 1 out]
                  n268 = global read "G_SEN.vi" "y_mobileye"() -> (w424:dbl[])
                  n269 = disable-structure shown="Enabled" {
                    disable-tunnel: w426 -> [w445 _]
                    disable-tunnel: w424 -> [w444 w446]
                    disable-tunnel: [w443 w446] -> w423
                    frame Disabled {
                      n270 = Array Subset(array=w444, length=w445) -> (w443:dbl[])  [unwired: 1 in]
                    }
                    frame Enabled {
                    }
                  }
                  n271 = Index Array(array=w425, index #1=1 ("index")) -> (element #1=w440:dbl, element #2=w439:dbl, element #3=w436:dbl)  [unwired: 2 in]
                  n272 = Multiply(x=w439, y=w423) -> (x*y=w437:dbl[])
                  n273 = Square(x=w423) -> (x^2=w441:dbl[])
                  n274 = Multiply(x=w440, y=w441) -> (x*y=w438:dbl[])
                  n275 = Compound Arithmetic op=ADD(w438, w437, w436) -> (w435:dbl[])
                }
              }
            }
          }
          "x 9" <- w381
          "y 9" <- w380
        }
        frame #10 {
          n276 = global read "G_SEN.vi" "Lane_L_M"() -> (w450:dbl[])
          n277 = Index Array(array=w450, index=0) -> (element=w448:dbl)
          n278 = Greater?(x=w448, y=0.65) -> (0:w449:bool)
          n279 = case shown="True" w449 {
            tunnel: w450 -> [_ w455]
            tunnel: [_ w456] -> w453
            tunnel: [_ w454] -> w452
            frame False {
            }
            frame True {
              n280 = global read "G_SEN.vi" "y_mobileye"() -> (w454:dbl[])
              n281 = Index Array(array=w455, index #1=1 ("index")) -> (element #1=w461:dbl, element #2=w460:dbl, element #3=w457:dbl)  [unwired: 2 in]
              n282 = Multiply(x=w460, y=w454) -> (x*y=w458:dbl[])
              n283 = Square(x=w454) -> (x^2=w462:dbl[])
              n284 = Multiply(x=w461, y=w462) -> (x*y=w459:dbl[])
              n285 = Compound Arithmetic op=ADD(w459, w458, w457) -> (w456:dbl[])
            }
          }
          "x 10" <- w453
          "y 10" <- w452
        }
        frame #11 {
          n286 = global read "G_SEN.vi" "Lane_R_M"() -> (w467:dbl[])
          n287 = Index Array(array=w467, index=0) -> (element=w465:dbl)
          n288 = Greater?(x=w465, y=0.65) -> (0:w466:bool)
          n289 = case shown="True" w466 {
            tunnel: w467 -> [_ w472]
            tunnel: [_ w473] -> w470
            tunnel: [_ w471] -> w469
            frame False {
            }
            frame True {
              n290 = global read "G_SEN.vi" "y_mobileye"() -> (w471:dbl[])
              n291 = Index Array(array=w472, index #1=1 ("index")) -> (element #1=w478:dbl, element #2=w477:dbl, element #3=w474:dbl)  [unwired: 2 in]
              n292 = Multiply(x=w477, y=w471) -> (x*y=w475:dbl[])
              n293 = Square(x=w471) -> (x^2=w479:dbl[])
              n294 = Multiply(x=w478, y=w479) -> (x*y=w476:dbl[])
              n295 = Compound Arithmetic op=ADD(w476, w475, w474) -> (w473:dbl[])
            }
          }
          "x 11" <- w470
          "y 11" <- w469
        }
        frame #12 {
          n296 = disable-structure shown="Enabled" {
            disable-tunnel: [w487 w490] -> w482
            disable-tunnel: [w486 w491] -> w481
            frame Disabled {
              n297 = disable-structure shown="Disabled" {
                disable-tunnel: [w488 w489 _] -> w485
                frame Disabled {
                  n298 = global read "G_SEN.vi" "sensor_etc"() -> (w488:dbl[][])
                }
                frame Enabled {
                  n299 = global read "G_SEN.vi" "sensor_temp"() -> (w489)
                }
                frame Disabled {
                  n300 = global read "G_SEN.vi" "sensor_obs_log"() -> ()  [unwired: 1 out]
                }
              }
              n301 = Index Array(array=w485, index (col) #1=0 ("disabled index (col)"), index (col) #2=1 ("index (col)")) -> (element #1=w486:dbl[], element #2=w487:dbl[])  [unwired: 2 in]
            }
            frame Enabled {
              n302 = global read "G_NAV.vi" "M6006"() -> (w494:T3)
              n303 = global read "G_SEN.vi" "sensor_obs_log"() -> (w499:dbl[][])
              n304 = Unbundle By Name(w494) -> ("lcc[1]"=w498:dbl, "lcc[0]"=w497:dbl, "attitude[2]"=w496:dbl)
              n305 = Negate(x=w496) -> (-x=w495:dbl)
              n306 = Index Array(array=w499, index (col) #1=0 ("disabled index (col)")) -> (element #1=w493:dbl[], element #2=w492:dbl[])  [unwired: 3 in]
              n307 = call "rotm_mimo.vi"("angle[rad]"=w495, "y0"=w497, "x0"=w498, "y"=w492, "x"=w493) -> ("Y"=w490:dbl[], "X"=w491:dbl[])  [unwired: 3 in, 2 out]
            }
          }
          "x 12" <- w481
          "y 12" <- w482
        }
        frame #13 {
          n308 = flat-sequence {
            tunnel: [w504] -> w502
            tunnel: [w503] -> w501
            frame #0 {
              n309 = global read "G_SEN.vi" "sensor_obs"() -> (w507:dbl[][])
              n310 = Index Array(array=w507, index (col) #1=0 ("disabled index (col)"), index (col) #2=1 ("index (col)")) -> (element #1=w506:dbl[], element #2=w505:dbl[])  [unwired: 2 in]
              n311 = disable-structure shown="Enabled" {
                disable-tunnel: w506 -> [w526 w528]
                disable-tunnel: w505 -> [w525 w527]
                disable-tunnel: [w511 w528] -> w504
                disable-tunnel: [w510 w527] -> w503
                frame Disabled {
                  n312 = global read "G_VEH.vi" "xsensor"() -> (w522:T4)
                  n313 = local read "M6006"() -> (w516:T1)
                  n314 = Unbundle By Name(w522) -> ("x"=w524:dbl, "y"=w523:dbl, "h"=w521:dbl)
                  n315 = Unbundle By Name(w516) -> ("lcc[1]"=w515:sgl, "lcc[0]"=w514:sgl, "attitude[2]"=w513:sgl)
                  n316 = Negate(x=w521) -> (-x=w520:dbl)
                  n317 = Negate(x=w513) -> (-x=w512:sgl)
                  n318 = call "rotm_mimo.vi"("angle[rad]"=w520, "reverse"=TRUE, "y0"=w523, "x0"=w524, "y"=w525, "x"=w526) -> ("Y"=w517:dbl[], "X"=w518:dbl[])  [unwired: 2 in, 2 out]
                  n319 = call "rotm_mimo.vi"("angle[rad]"=w512, "y0"=w514, "x0"=w515, "y"=w517, "x"=w518) -> ("Y"=w510:dbl[], "X"=w511:dbl[])  [unwired: 3 in, 2 out]
                }
                frame Enabled {
                }
              }
            }
          }
          "x 13" <- w502
          "y 13" <- w501
        }
        frame #14 {
          n320 = disable-structure shown="Enabled" {
            disable-tunnel: [w531 w536 w552] -> w529
            disable-tunnel: [w532 w535 w551] -> w530
            frame Disabled {
              n321 = global read "G_SEN.vi" "sensor_lane"() -> (w533:dbl[][])
              n322 = Index Array(array=w533, index (col) #1=0 ("disabled index (col)")) -> (element #1=w532:dbl[], element #2=w531:dbl[])  [unwired: 3 in]
            }
            frame Enabled {
              n323 = global read "G_NAV.vi" "M6006"() -> (w539:T3)
              n324 = global read "G_SEN.vi" "sensor_lane_log"() -> (w544:dbl[][])
              n325 = Unbundle By Name(w539) -> ("lcc[1]"=w543:dbl, "lcc[0]"=w542:dbl, "attitude[2]"=w541:dbl)
              n326 = Negate(x=w541) -> (-x=w540:dbl)
              n327 = Index Array(array=w544, index (col) #1=0 ("disabled index (col)")) -> (element #1=w538:dbl[], element #2=w537:dbl[])  [unwired: 3 in]
              n328 = call "rotm_mimo.vi"("angle[rad]"=w540, "y0"=w542, "x0"=w543, "y"=w537, "x"=w538) -> ("Y"=w536:dbl[], "X"=w535:dbl[])  [unwired: 3 in, 2 out]
            }
            frame Disabled {
              n329 = global read "G_SEN.vi" "lane_log_RR"() -> (w546:dbl[][])
              n330 = global read "G_SEN.vi" "lane_log_LL"() -> (w547:dbl[][])
              n331 = global read "G_SEN.vi" "lane_log_L"() -> (w550:dbl[][])
              n332 = global read "G_SEN.vi" "lane_log_R"() -> (w549:dbl[][])
              n333 = global read "G_NAV.vi" "M6006"() -> (w555:T3)
              n334 = Unbundle By Name(w555) -> ("lcc[1]"=w559:dbl, "lcc[0]"=w558:dbl, "attitude[2]"=w557:dbl)
              n335 = Build Array (concatenate)(w547, w550, w549, w546) -> (w548:dbl[][])
              n336 = Negate(x=w557) -> (-x=w556:dbl)
              n337 = Index Array(array=w548, index (col) #1=0 ("disabled index (col)")) -> (element #1=w554:dbl[], element #2=w553:dbl[])  [unwired: 3 in]
              n338 = call "rotm_mimo.vi"("angle[rad]"=w556, "y0"=w558, "x0"=w559, "y"=w553, "x"=w554) -> ("Y"=w552:dbl[], "X"=w551:dbl[])  [unwired: 3 in, 2 out]
            }
          }
          "x 14" <- w530
          "y 14" <- w529
        }
        frame #15 {
          n339 = flat-sequence {
            tunnel: [w564] -> w562
            tunnel: [w563] -> w561
            frame #0 {
              n340 = global read "G_VEH.vi" "xsensor"() -> (w575:T4)
              n341 = global read "G_SEN.vi" "sensor_lane"() -> (w580:dbl[][])
              n342 = local read "M6006"() -> (w569:T1)
              n343 = Unbundle By Name(w575) -> ("x"=w577:dbl, "y"=w576:dbl, "h"=w574:dbl)
              n344 = Unbundle By Name(w569) -> ("lcc[1]"=w568:sgl, "lcc[0]"=w567:sgl, "attitude[2]"=w566:sgl)
              n345 = Negate(x=w574) -> (-x=w573:dbl)
              n346 = Index Array(array=w580, index (col) #1=0 ("disabled index (col)"), index (col) #2=1 ("index (col)")) -> (element #1=w579:dbl[], element #2=w578:dbl[])  [unwired: 2 in]
              n347 = Negate(x=w566) -> (-x=w565:sgl)
              n348 = call "rotm_mimo.vi"("angle[rad]"=w573, "reverse"=TRUE, "y0"=w576, "x0"=w577, "y"=w578, "x"=w579) -> ("Y"=w570:dbl[], "X"=w571:dbl[])  [unwired: 2 in, 2 out]
              n349 = call "rotm_mimo.vi"("angle[rad]"=w565, "y0"=w567, "x0"=w568, "y"=w570, "x"=w571) -> ("Y"=w563:dbl[], "X"=w564:dbl[])  [unwired: 3 in, 2 out]
            }
          }
          "x 15" <- w562
          "y 15" <- w561
        }
        frame #16 {
          "x 16" <- dbl[] [-0.925, -0.925, -0.925, -0.6775, -0.6775, -0.925, -0.925, -0.925, -0.925, -0.6775, -0.6775, -0.925, -0.925, -0.925, 0.9025, 0.9025, 0.9025, 0.6775, 0.6775, 0.9025, 0.9025, 0.9025, 0.9025, 0.6775, 0.6775, 0.9025, 0.9025, 0.9025, -0.925] ("car_x")
          "y 16" <- dbl[] [-0.75, -0.224, 0.224, 0.224, -0.224, -0.224, 0.224, 2.415, 2.885, 2.885, 2.415, 2.415, 2.885, 3.5, 3.5, 2.885, 2.415, 2.415, 2.885, 2.885, 2.415, 0.224, -0.224, -0.224, 0.224, 0.224, -0.224, -0.75, -0.75] ("car_y")
        }
        frame #17 {
          n350 = disable-structure shown="Enabled" {
            disable-tunnel: [w590 w591] -> w588
            disable-tunnel: [1 ("disabled index (col)") _] -> w587
            frame Disabled {
              n351 = global read "G_SEN.vi" "sensor_velodyne"() -> (w590)
            }
            frame Enabled {
              n352 = global read "G_SEN.vi" "sensor_velodyne_chopped"() -> (w591:dbl[][])
            }
          }
          n353 = Index Array(array=w588, index (col) #1=w587) -> (element #1=→"x 17":dbl[], element #2=→"y 17":dbl[])  [unwired: 3 in]
        }
      }
    }
    frame #1 {
      n354 = flat-sequence {
        tunnel: [w627] -> w593
        frame #0 {
          n355 = local read "x 10"() -> (w619:dbl[])
          n356 = local read "x 11"() -> (w615:dbl[])
          n357 = local read "x 12"() -> (w613:dbl[])
          n358 = local read "x 13"() -> (w611:dbl[])
          n359 = local read "x 14"() -> (w608:dbl[])
          n360 = local read "x 15"() -> (w610:dbl[])
          n361 = local read "x 16"() -> (w597:dbl[])
          n362 = local read "x 17"() -> (w596:dbl[])
          n363 = local read "x 1"() -> (w629:dbl[])
          n364 = local read "x 2"() -> (w626:dbl[])
          n365 = local read "x 3"() -> (w624:dbl[])
          n366 = local read "x 4"() -> (w601:dbl[])
          n367 = local read "x 5"() -> (w599:dbl[])
          n368 = local read "x 6"() -> (w622:dbl[])
          n369 = local read "x 7"() -> (w621:dbl[])
          n370 = local read "x 8"() -> (w616:dbl[])
          n371 = local read "x 9"() -> (w618:dbl[])
          n372 = call "Convert to Dynamic Data9"("Array"=w619) -> ("Dynamic Data Type"=w607:dynamicdata)  [unwired: 3 in]
          n373 = call "Convert to Dynamic Data17"("Array"=w615) -> ("Dynamic Data Type"=w614:dynamicdata)  [unwired: 3 in]
          n374 = call "Convert to Dynamic Data18"("Array"=w613) -> ("Dynamic Data Type"=w612:dynamicdata)  [unwired: 3 in]
          n375 = call "Convert to Dynamic Data21"("Array"=w611) -> ("Dynamic Data Type"=w609:dynamicdata)  [unwired: 3 in]
          n376 = call "Convert to Dynamic Data26"("Array"=w608) -> ("Dynamic Data Type"=w602:dynamicdata)  [unwired: 3 in]
          n377 = call "Convert to Dynamic Data22"("Array"=w610) -> ("Dynamic Data Type"=w603:dynamicdata)  [unwired: 3 in]
          n378 = call "Convert to Dynamic Data24"("Array"=w597) -> ("Dynamic Data Type"=w604:dynamicdata)  [unwired: 3 in]
          n379 = call "Convert to Dynamic Data34"("Array"=w596) -> ("Dynamic Data Type"=w595:dynamicdata)  [unwired: 3 in]
          n380 = call "Convert to Dynamic Data"("Array"=w629) -> ("Dynamic Data Type"=w628:dynamicdata)  [unwired: 3 in]
          n381 = call "Convert to Dynamic Data3"("Array"=w626) -> ("Dynamic Data Type"=w625:dynamicdata)  [unwired: 3 in]
          n382 = call "Convert to Dynamic Data5"("Array"=w624) -> ("Dynamic Data Type"=w623:dynamicdata)  [unwired: 3 in]
          n383 = call "Convert to Dynamic Data29"("Array"=w601) -> ("Dynamic Data Type"=w600:dynamicdata)  [unwired: 3 in]
          n384 = call "Convert to Dynamic Data31"("Array"=w599) -> ("Dynamic Data Type"=w598:dynamicdata)  [unwired: 3 in]
          n385 = call "Convert to Dynamic Data27"("Array"=w622) -> ("Dynamic Data Type"=w605:dynamicdata)  [unwired: 3 in]
          n386 = call "Convert to Dynamic Data7"("Array"=w621) -> ("Dynamic Data Type"=w620:dynamicdata)  [unwired: 3 in]
          n387 = call "Convert to Dynamic Data14"("Array"=w616) -> ("Dynamic Data Type"=w606:dynamicdata)  [unwired: 3 in]
          n388 = call "Convert to Dynamic Data11"("Array"=w618) -> ("Dynamic Data Type"=w617:dynamicdata)  [unwired: 3 in]
          n389 = Merge Signals(w628, w625, w623, w600, w598, w605, w620, w606, w617, w607, w614, w612, w609, w602, w603, w604, w595) -> (w627:dynamicdata)
        }
      }
      n390 = flat-sequence {
        tunnel: [w662] -> w592
        frame #0 {
          n391 = local read "y 10"() -> (w654:dbl[])
          n392 = local read "y 11"() -> (w650:dbl[])
          n393 = local read "y 12"() -> (w648:dbl[])
          n394 = local read "y 13"() -> (w646:dbl[])
          n395 = local read "y 14"() -> (w643:dbl[])
          n396 = local read "y 15"() -> (w644:dbl[])
          n397 = local read "y 16"() -> (w632:dbl[])
          n398 = local read "y 17"() -> (w631:dbl[])
          n399 = local read "y 1"() -> (w664:dbl[])
          n400 = local read "y 2"() -> (w661:dbl[])
          n401 = local read "y 3"() -> (w659:dbl[])
          n402 = local read "y 4"() -> (w636:dbl[])
          n403 = local read "y 5"() -> (w634:dbl[])
          n404 = local read "y 6"() -> (w657:dbl[])
          n405 = local read "y 7"() -> (w656:dbl[])
          n406 = local read "y 8"() -> (w651:dbl[])
          n407 = local read "y 9"() -> (w653:dbl[])
          n408 = call "Convert to Dynamic Data10"("Array"=w654) -> ("Dynamic Data Type"=w642:dynamicdata)  [unwired: 3 in]
          n409 = call "Convert to Dynamic Data15"("Array"=w650) -> ("Dynamic Data Type"=w649:dynamicdata)  [unwired: 3 in]
          n410 = call "Convert to Dynamic Data16"("Array"=w648) -> ("Dynamic Data Type"=w647:dynamicdata)  [unwired: 3 in]
          n411 = call "Convert to Dynamic Data19"("Array"=w646) -> ("Dynamic Data Type"=w645:dynamicdata)  [unwired: 3 in]
          n412 = call "Convert to Dynamic Data25"("Array"=w643) -> ("Dynamic Data Type"=w637:dynamicdata)  [unwired: 3 in]
          n413 = call "Convert to Dynamic Data20"("Array"=w644) -> ("Dynamic Data Type"=w638:dynamicdata)  [unwired: 3 in]
          n414 = call "Convert to Dynamic Data23"("Array"=w632) -> ("Dynamic Data Type"=w639:dynamicdata)  [unwired: 3 in]
          n415 = call "Convert to Dynamic Data33"("Array"=w631) -> ("Dynamic Data Type"=w630:dynamicdata)  [unwired: 3 in]
          n416 = call "Convert to Dynamic Data2"("Array"=w664) -> ("Dynamic Data Type"=w663:dynamicdata)  [unwired: 3 in]
          n417 = call "Convert to Dynamic Data4"("Array"=w661) -> ("Dynamic Data Type"=w660:dynamicdata)  [unwired: 3 in]
          n418 = call "Convert to Dynamic Data6"("Array"=w659) -> ("Dynamic Data Type"=w658:dynamicdata)  [unwired: 3 in]
          n419 = call "Convert to Dynamic Data30"("Array"=w636) -> ("Dynamic Data Type"=w635:dynamicdata)  [unwired: 3 in]
          n420 = call "Convert to Dynamic Data32"("Array"=w634) -> ("Dynamic Data Type"=w633:dynamicdata)  [unwired: 3 in]
          n421 = call "Convert to Dynamic Data28"("Array"=w657) -> ("Dynamic Data Type"=w640:dynamicdata)  [unwired: 3 in]
          n422 = call "Convert to Dynamic Data8"("Array"=w656) -> ("Dynamic Data Type"=w655:dynamicdata)  [unwired: 3 in]
          n423 = call "Convert to Dynamic Data13"("Array"=w651) -> ("Dynamic Data Type"=w641:dynamicdata)  [unwired: 3 in]
          n424 = call "Convert to Dynamic Data12"("Array"=w653) -> ("Dynamic Data Type"=w652:dynamicdata)  [unwired: 3 in]
          n425 = Merge Signals(w663, w660, w658, w635, w633, w640, w655, w641, w652, w642, w649, w647, w645, w637, w638, w639, w630) -> (w662:dynamicdata)
        }
      }
      n426 = call "GRAPH"("Y Input"=w592, "X Input"=w593) -> ("XY Graph"=→"XY Graph":cluster{"Y":dbl[], "Y":dbl[]}[])  [unwired: 3 in, 6 out]
    }
  }
